vi "Main.vi"() -> ()   [LabVIEW 2021]
uses:
  Hamamatsu_class/SubRegion.ctl
  Application_class/Application.lvclass
  CetoniPump_class/CetoniPump.lvclass
  <vilib>/vision/Image Controls.llb/IMAQ Image.ctl
  Coriolis_Sim_class/Coriolis_Sim.lvclass
  C:/GIT/DensityGradientProject/CoriFlowBFS1Plus_class/CoriFlowBFS1Plus.lvclass
  CoriFlowBFS1Plus_class/CoriFlowBFS1Plus.lvclass
  Experiment_class/Experiment.lvclass
  <vilib>/Utility/error.llb/Error Cluster From Error Code.vi
  <vilib>/ErrorRing/Error Ring.xnode
  AD2_SDK_class/AD2_SDK.lvclass
  Hamamatsu_class/Hamamatsu.lvclass
panel:
  in  "Part of Experiment":bool
  in  "Numeric":dbl
  out "Configured Syringes":T1(array[cluster])
  in  "ABORT":bool
  out "Status":string="Cetoni Pump Initialized"
  out "Connected Pumps":T2(array[cluster])
  out "error out":errorcluster={"status"=TRUE, "code"=-2, "source"="labbCAN_Bus_API.lvlib:Error Converter (ErrCode or Status).vi<ERR>\nNo such entity\r\nThe given device config directory [C:\\Users\\Public\\Documents\\QmixElements\\Projects\\default_project\\Configurations] does not contain the required file device_properties.xml.\n\n\n<b>Complete call chain:</b>\r\n     labbCAN_Bus_API.lvlib:Error Converter (ErrCode or Status).vi\r\n     labbCAN_Bus_API.lvlib:LCB Open.vi\r\n     CetoniPump.lvclass:CetoniPump_Init.vi\r\n     Main.vi"}
  in  "Tab Control":T3(tab)=enum."LOG"
  in  "Connect TO Hardware":bool
  in  "Filter(0-1)Min-Max":dbl=0.5 min=0.0 max=1.0
  in  "Coriolis VISA resource name":refnum<visa-resource-name>="COM3"
  in  "Use Coriolis?":bool=TRUE
  in  "Cetoni Configuration Path":string="C:\\Users\\Public\\Documents\\QmixElements\\Projects\\default_project\\Configurations\\Gradient_generator_2"
  in  "Load and set latest":bool
  in  "Read Current Syringe \nConfiguration":bool
  in  "Read Continous":bool
  in  "Go to Level":bool
  in  "Go to Level":T4
  in  "index":i32
  in  "ReferenceMove":bool
  in  "ReadStatus":bool
  in  "ConfigureSyringe":bool
  in  "SyringeSettings":T5={"index"=0, "SyringeSettings"={"Maximum Piston Stroke (mm)"=100.0, "Inner Diameter (mm)"=12.0}}
  in  "Syringe (only for syringe helper)":T6(ring)=enum."BD 5ml"
  out "Syringe Helper":T7={"Maximum Piston Stroke (mm)"=48.147993421803335, "Inner Diameter (mm)"=12.06}
  in  "Stop ALL Pumps":bool
  in  "CetoniWaitData":T8
  in  "Cetoni Wait for Level":bool
  in  "Save Current Configuration":bool
  in  "Ramp IN flow":bool
  in  "Ramp In Settings":T9
  in  "Open Image Pairs Windows":bool
  in  "Open Live Window":bool
  in  "Center ROI":bool
  in  "Configure ROI":bool
  in  "ROI":T10={"Horizontal Offset"=0, "Vertical Offset"=0, "Horizontal Size"=2048, "Vertical Size"=2048} {"Vertical Size" min=4 max=2304 step=4; "Horizontal Size" min=4 max=2304 step=4; "Vertical Offset" min=0 max=0 step=4; "Horizontal Offset" min=0 max=0 step=4}
  in  "Go Live":bool
  in  "Set Exposure Time":bool
  in  "Read Redout Time":bool
  out "ReadoutTime":dbl
  in  "Exposure (ms)":dbl=5.0 step=1.0
  in  "Take HW Timed Image Pair":bool
  in  "Save HW Timed Image Pair":bool
  in  "Image Continously":bool
  in  "Configure Triggering":bool
  in  "Open DIO signal helper":bool
  in  "Triggering":T11={"Pulse Length(ms)"=10.0, "DIO0Offset(ms)"=0.0, "DIO1 Pulse time (ms)"=10.0, "DIO2 Pulse time (ms) 2"=100.0, "DIO3 Pulse time (ms) 3"=0.0, "EnableDIO3"=FALSE, "EnableDIO2"=TRUE, "EnableDIO1"=TRUE}
  out "Waveform Chart":T12(graph)
  in  "Read Continously?":bool
  in  "Read Coriolis":bool
  in  "Read Coriolis Buffer":bool
  out "Buffer":T13(array[cluster])
  out "Coriolis  Data":T14
  in  "Wait":bool
  in  "Wait":T15={"Wait Time"=0.0, "Reset"=FALSE, "Part of Experiment"=TRUE}
  in  "Read Trigges Values From HW Timed TAB":bool
  in  "Run Experiment":bool
  in  "Create Experiment":bool
  in  "Experiment Base path":path
  in  "Number of Images at each Level":u16
  in  "Levels (uL)":dbl[](array[numeric])
  in  "Triggering for experiment":T11
  in  "Ramp In (Experiment)":T9
  out "LOG":string
  in  "Exit":bool
  in  "Inject Error<Replace Me>":bool
  # "Not implemented"
  # "DIO0 Pulses at the same time as DIO1,2 and 3 +-offset"
  # "DIO0 Pulses at the same time as DIO1,2 \nand 3 +-offset"
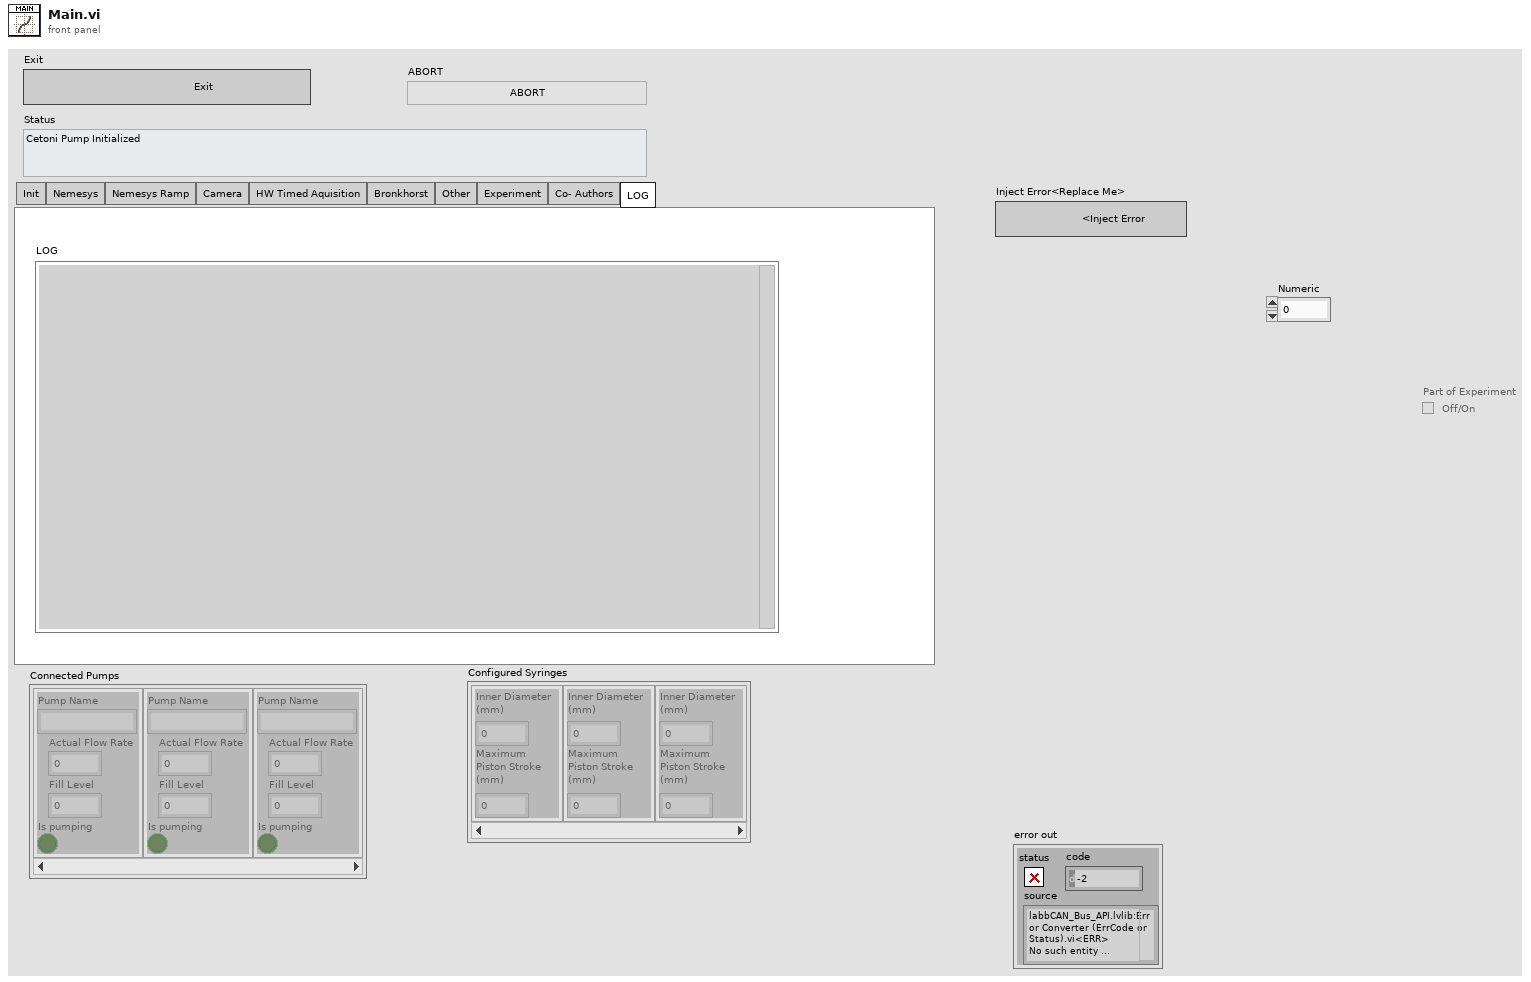
[diagram p1: front panel]
types:
  T1 = cluster{"Inner Diameter \n(mm)":dbl, "Maximum \nPiston Stroke \n(mm)":dbl}[]
  T2 = cluster{"Pump Name":string, "Actual Flow Rate":dbl, "Fill Level":dbl, "Is pumping":bool}[]
  T3 = enum32{"Init", "Nemesys", "Nemesys Ramp", "Camera", "HW Timed Aquisition", "Bronkhorst", "Other", "Experiment", "Co- Authors", "LOG"}
  T4 = cluster{"index":i32, "Flow (ul/min)":dbl, "Level(uL)":dbl}
  T5 = cluster{"index":i32, "SyringeSettings":cluster{"Maximum Piston Stroke (mm)":dbl, "Inner Diameter (mm)":dbl}}
  T6 = enum16{"BD 1ml", "BD 3ml", "BD 5ml", "BD 10ml", "BD 20ml", "BD 30ml", "BD 50ml", "HSW 1ml"}
  T7 = cluster{"Maximum Piston Stroke (mm)":dbl, "Inner Diameter (mm)":dbl}
  T8 = cluster{"Index":u8, "WaitCondition":enum16{"GE", "LE", "Stopped"}, "Value (uL)":dbl, "Experiment":bool}
  T9 = cluster{"Pump Controller":cluster{"Index of Pump Controller":u8, "Medium Start Before  Level (uL))":dbl, "Slow Start Before  Level (uL)":dbl, "Target Level (uL)":dbl}, "Pump Flows":cluster{"Index of Pump":u8, "Fast Flow":dbl, "Medium Flow":dbl, "Slow Flow":dbl}[]}
  T10 = typedef "Hamamatsu.lvclass/SubRegion.ctl" = cluster{"Horizontal Offset":i32, "Vertical Offset":i32, "Horizontal Size":i32, "Vertical Size":i32}
  T11 = cluster{"Pulse Length(ms)":dbl, "DIO0Offset(ms)":dbl, "DIO1 Pulse time (ms)":dbl, "DIO2 Pulse time (ms) 2":dbl, "DIO3 Pulse time (ms) 3":dbl, "EnableDIO3":bool, "EnableDIO2":bool, "EnableDIO1":bool}
  T12 = cluster{"Density_g_L":sgl, "FLow(ul/min)":sgl, "Temperature(C)":sgl}
  T13 = cluster{"Cluster":cluster{"Density_g_L":sgl, "FLow(ul/min)":sgl, "Temperature(C)":sgl}, "current time":timestamp}[]
  T14 = cluster{"Cluster":cluster{"Density_g_L":sgl, "FLow(ul/min)":sgl, "Temperature(C)":sgl}, "current time":timestamp}
  T15 = cluster{"Wait Time":dbl, "Reset":bool, "Part of Experiment":bool}
  T16 = enum8{"Enabled", "Disabled", "Disabled and Grayed Out"}
  T17 = cluster{"Index":u8, "WaitCondition":enum16{"GE", "LE", "Stopped"}, "Value":dbl, "Experiment":bool}
  T18 = cluster{"Pump Handle":i64, "Pump Name":string, "Maximum Volume":dbl, "Maximum Flow Rate":dbl, "Flow Rate":dbl, "Target Level":dbl}[]
  T19 = cluster{"Inner Diameter (mm)":dbl, "Maximum Piston Stroke (mm)":dbl}[]
  T20 = cluster{"Ramp In Settings":cluster{"Pump Controller":cluster{"Index of Pump Controller":u8, "Medium Start Before  Level (uL))":dbl, "Slow Start Before  Level (uL)":dbl, "Target Level (uL)":dbl}, "Pump Flows":cluster{"Index of Pump":u8, "Fast Flow":dbl, "Medium Flow":dbl, "Slow Flow":dbl}[]}, bool}
  T21 = cluster{"Fill Level":dbl, "Is pumping":bool, "Actual Flow Rate":dbl}
  T22 = typedef "IMAQ Image.ctl" = refnum<image>
  T23 = typedef "LVMinMaxIncTypeDef.ctl" = cluster{"Minimum":dbl, "Maximum":dbl, "Increment":dbl}
  T24 = cluster{"H Offset":cluster{"Value":i32, "Limits":T23}, "V Offset":cluster{"Value":i32, "Limits":T23}, "H Size":cluster{"Value":i32, "Limits":T23}, "V Size":cluster{"Value":i32, "Limits":T23}}
  T25 = typedef "Hamamatsu.lvclass/SubRegionLimits.ctl" = cluster{"H Offset":cluster{"Value":i32, "Limits":T23}, "V Offset":cluster{"Value":i32, "Limits":T23}, "H Size":cluster{"Value":i32, "Limits":T23}, "V Size":cluster{"Value":i32, "Limits":T23}}
  T26 = enum32{"Invalid", "Standard", "Closed", "Hidden", "Minimized", "Maximized"}
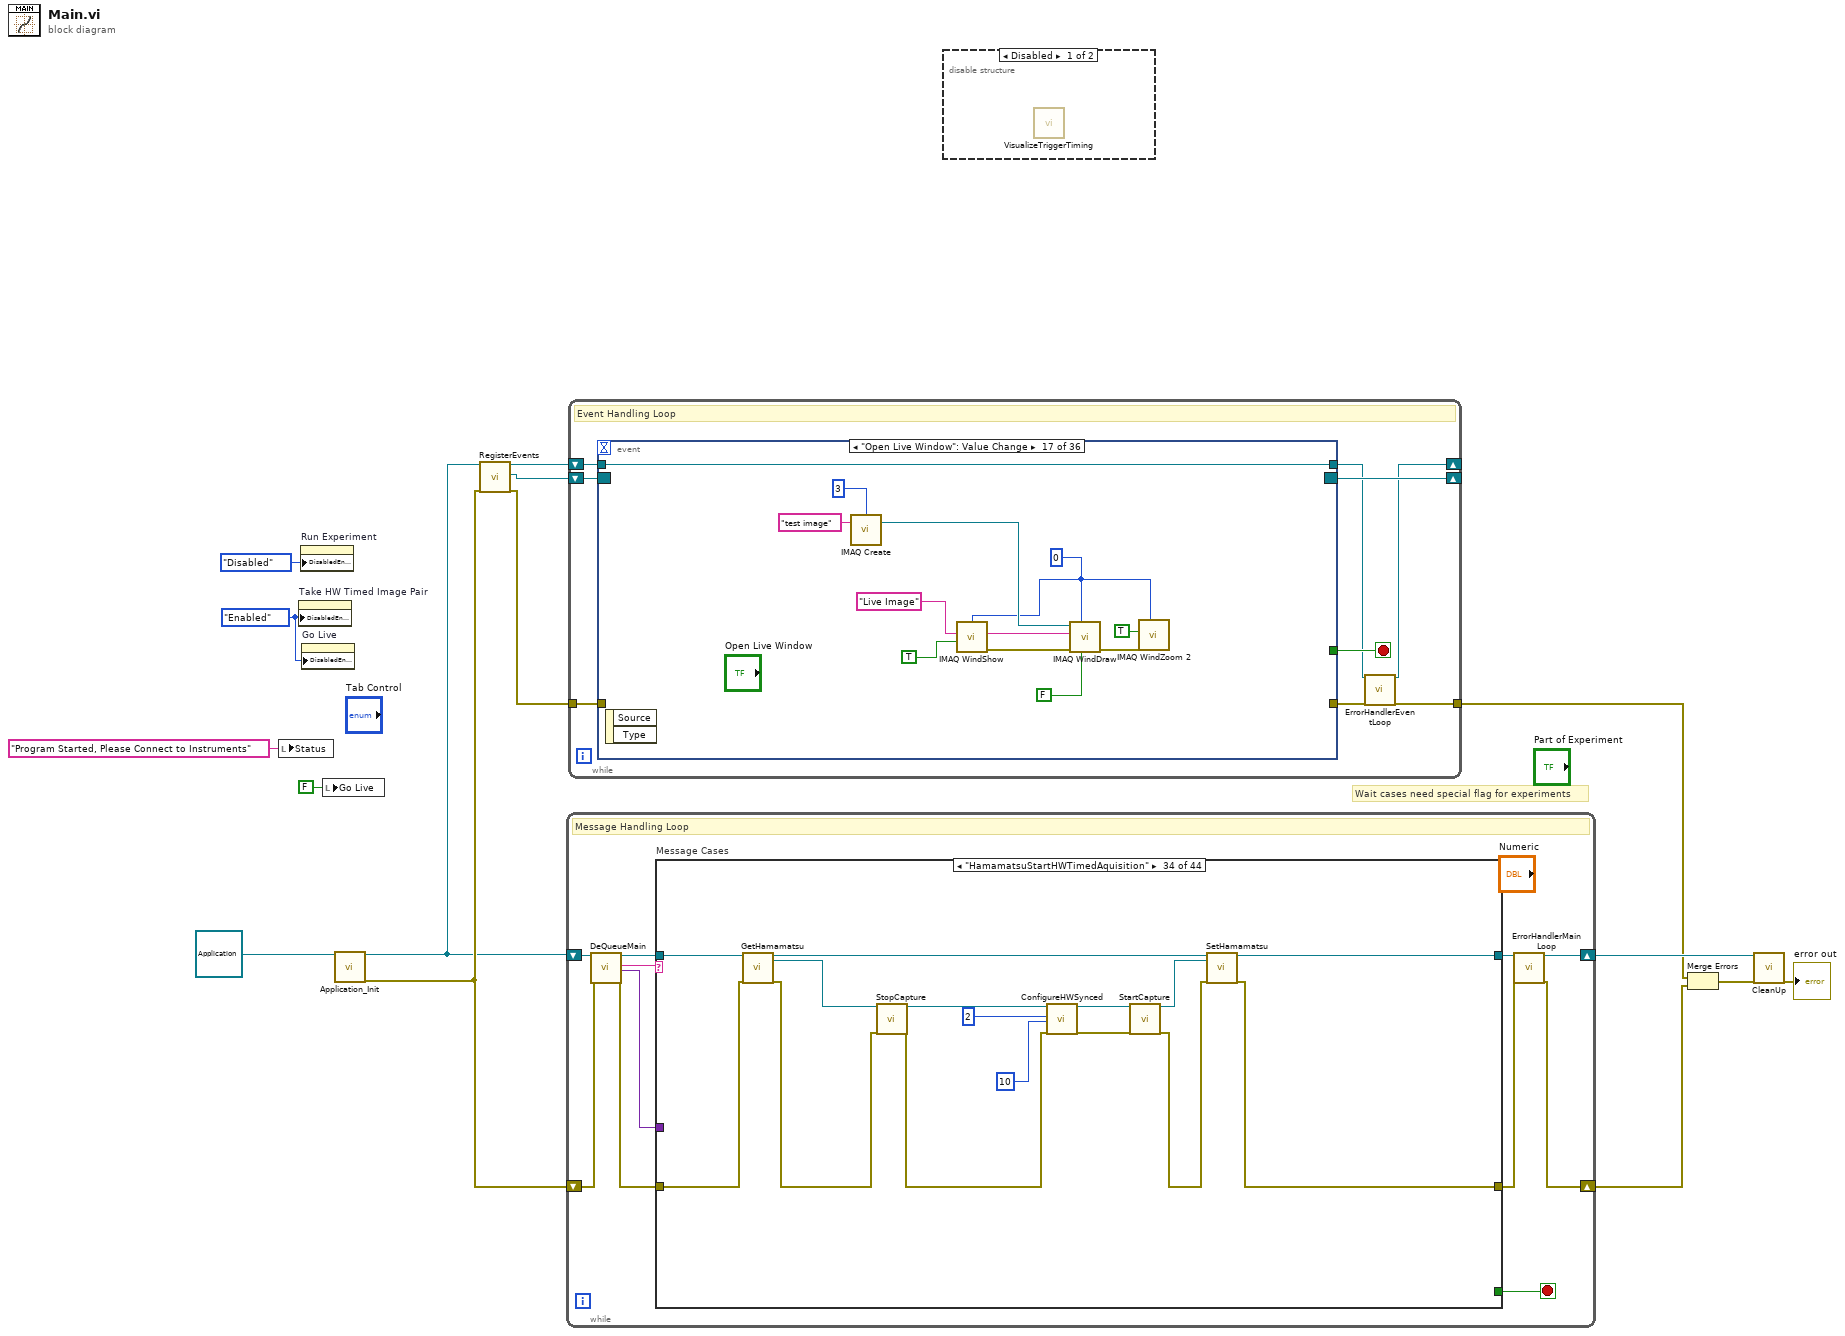
[diagram p0: block diagram]
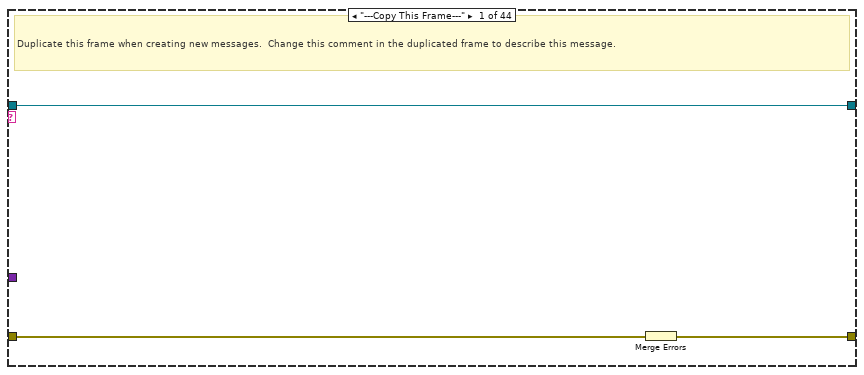
[diagram p3: hidden frame]
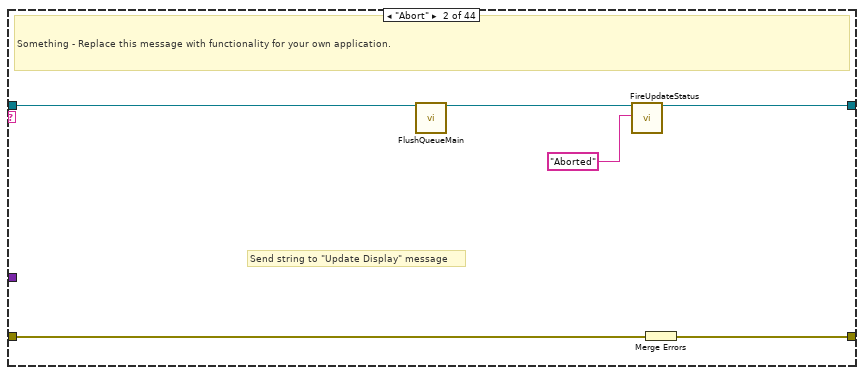
[diagram p4: hidden frame]
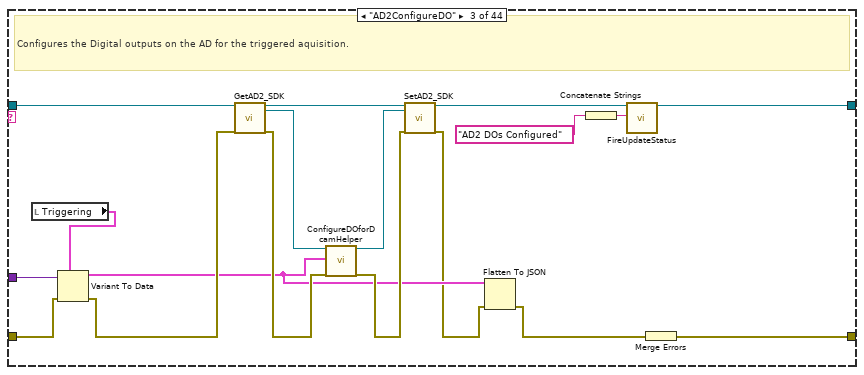
[diagram p5: hidden frame]
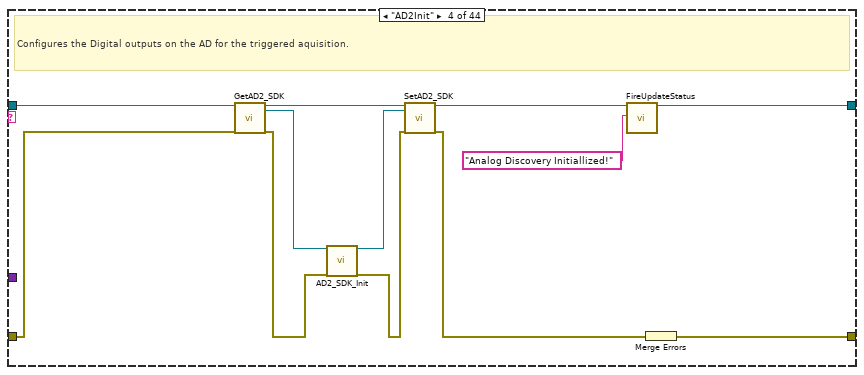
[diagram p6: hidden frame]
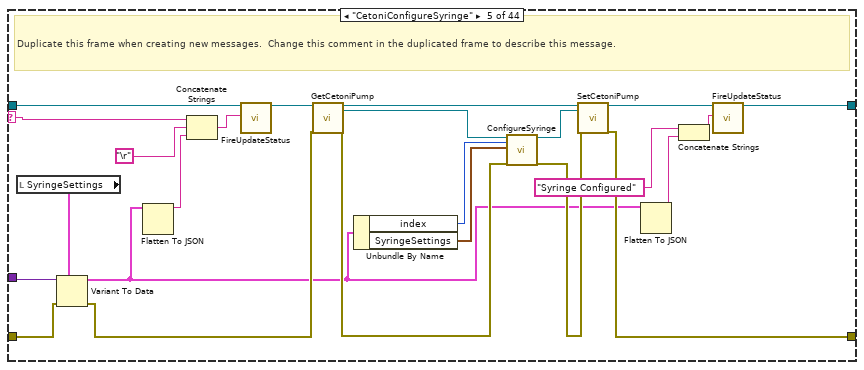
[diagram p7: hidden frame]
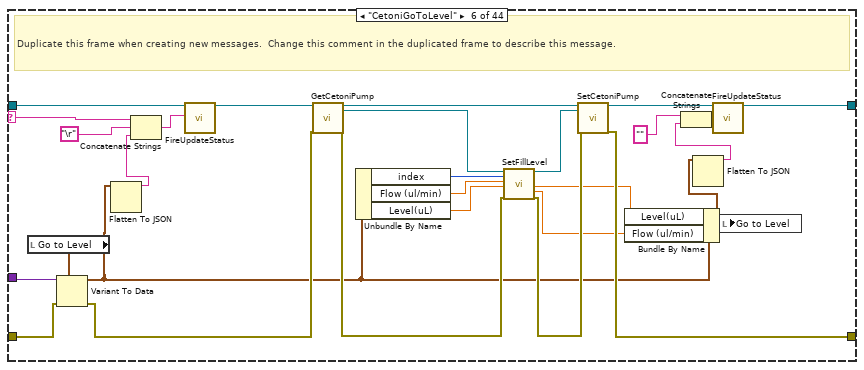
[diagram p8: hidden frame]
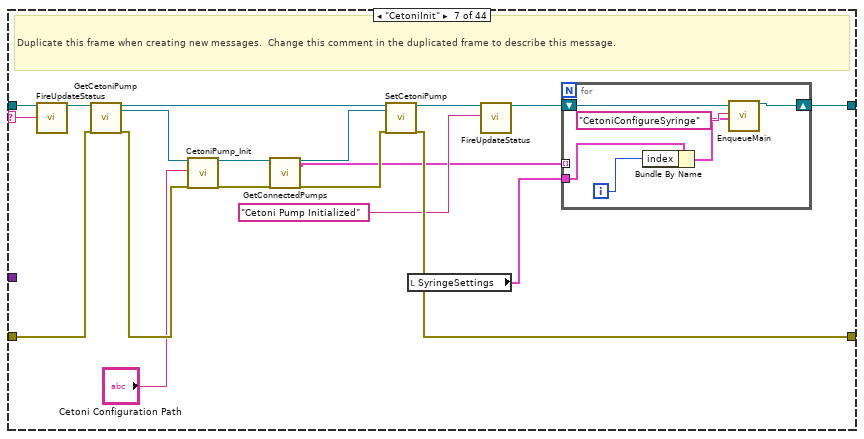
[diagram p9: hidden frame]
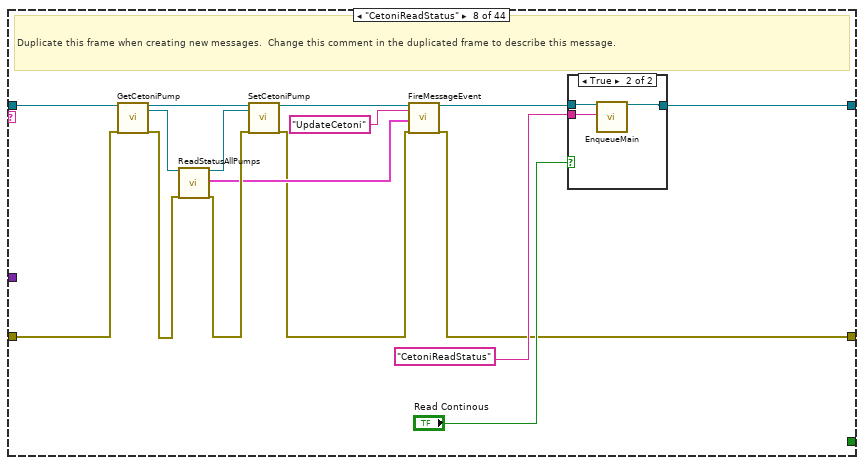
[diagram p10: hidden frame]
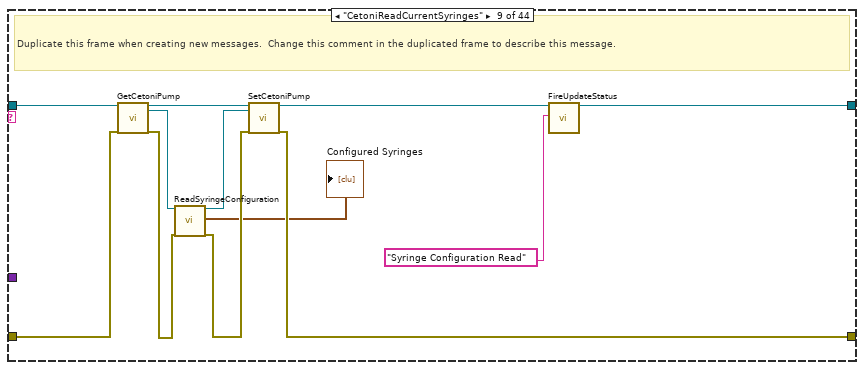
[diagram p12: hidden frame]
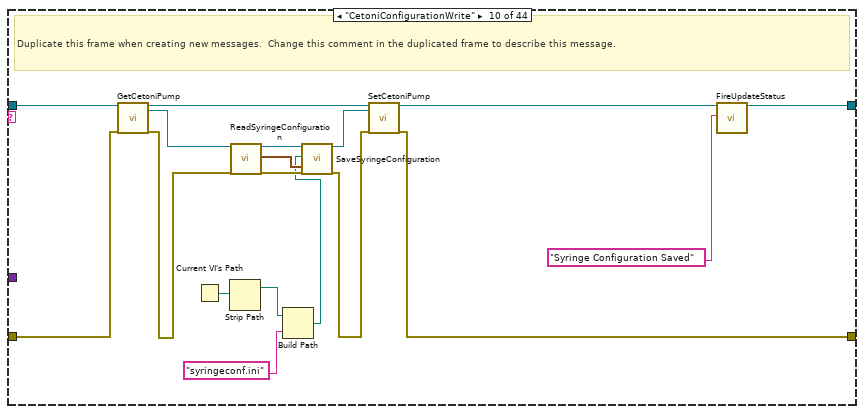
[diagram p13: hidden frame]
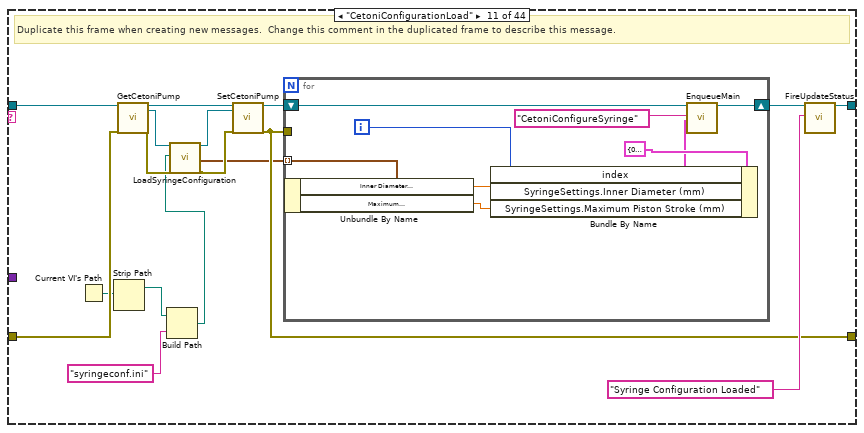
[diagram p14: hidden frame]
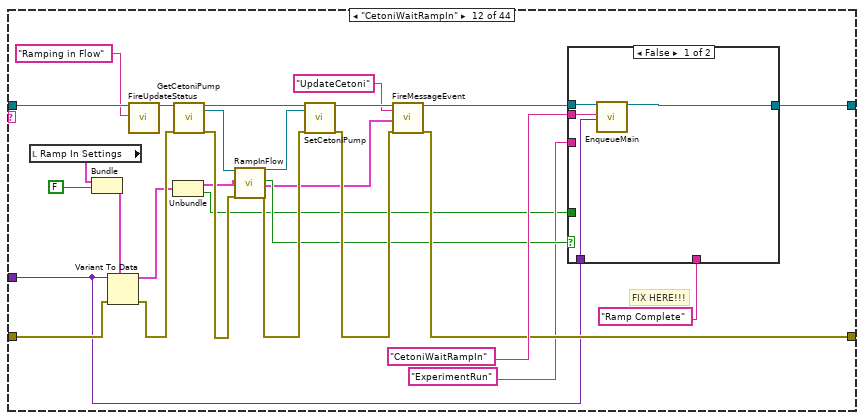
[diagram p15: hidden frame]
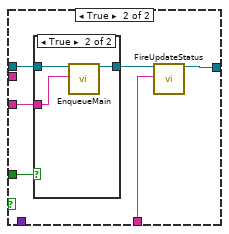
[diagram p16: hidden frame]
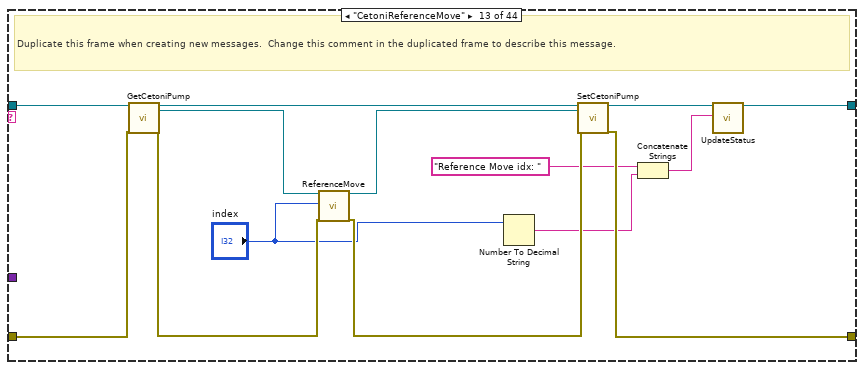
[diagram p18: hidden frame]
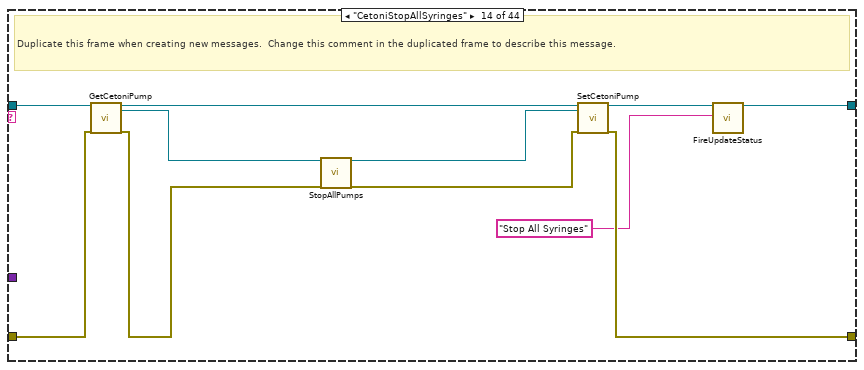
[diagram p19: hidden frame]
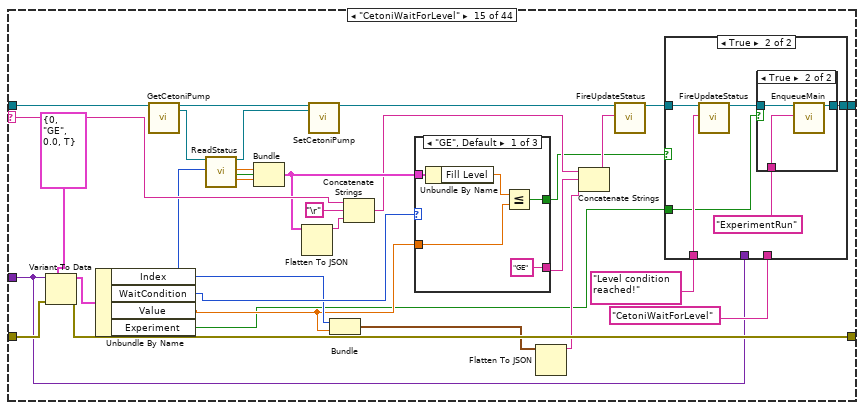
[diagram p20: hidden frame]
diagram:
  w3 = T16."Enabled" ("Disabled")
  # "Wait cases need special flag for experiments"
  n1 = local write "Status"("Program Started, Please Connect to Instruments" ("Status")) -> ()
  n2 = property on="Take HW Timed Image Pair" class="Bool"("DisabledEnum"=w3) -> ()  [unwired: 2 in, 2 out]
  n3 = property on="Run Experiment" class="Bool"("DisabledEnum"=T16."Disabled" ("Disabled")) -> ()  [unwired: 2 in, 2 out]
  n4 = property on="Go Live" class="Bool (strict)"("DisabledEnum"=w3) -> ()  [unwired: 2 in, 2 out]
  n5 = local write "Go Live"(FALSE ("Go Live")) -> ()
  n6 = call "Application_Init.vi"("object in"=refnum<class "Application.lvclass"> refnum ("Application")) -> ("object out"=w5:refnum<class "Application.lvclass">, "error out"=w11:errorcluster)  [unwired: 17 in]
  n7 = call-dynamic "RegisterEvents.vi"("object in"=w5, "error in (no error)"=w11) -> ("object out"=w13:refnum<class "Application.lvclass">, "Event Registration Refnum"=w14:refnum<event-registration>, "error out"=w12:errorcluster)  [unwired: 15 in]
  n8 = while {
    shift-right: [w19] -> w10
    shift-left: w5 -> [w25]
    shift-right: [w20] -> w9
    shift-left: w11 -> [w16]
    stop <- w26 stop-if-true
    # "Message Handling Loop"
    n9 = call-dynamic "DeQueueMain.vi"("object in"=w25, "error in (no error)"=w16) -> ("object out"=w24:refnum<class "Application.lvclass">, "Message"=w23:string, "Message Data"=w22:variant, "error out"=w17:errorcluster)  [unwired: 14 in]
    n10 = case "Message Cases" shown="\"HamamatsuStartHWTimedAquisition\"" w23 {
      selector: w23 -> [_ _ _ _ w73 w103 w127 _ _ _ _ _ _ _ w311 _ _ _ _ _ _ _ _ _ _ _ _ _ _ _ _ w637 _ _ _ _ _ _ _ _ _ _ _ w872]
      tunnel: w17 -> [w29 w34 w43 w60 w84 w105 w134 w156 w172 w190 w207 w229 w270 w283 w306 w350 w361 w381 w401 w408 w417 w430 w432 w439 w466 w491 w507 w548 w571 w584 w616 w653 w662 w676 w693 w704 w731 w760 w765 w776 w814 w831 w843 _]
      tunnel: [w28 w35 w53 w65 w88 w115 w129 w143 w170 w188 w194 w236 w272 w281 w307 w349 w367 w393 w407 w409 w423 w425 w433 w448 w459 w491 w508 w554 w575 w583 w608 w652 w661 w674 w686 w702 w734 w760 w770 w797 w812 w832 w843 w873] -> w21
      tunnel: [_ _ _ _ _ _ _ _ _ _ _ _ _ _ _ _ _ _ _ _ _ _ TRUE _ _ _ _ _ _ _ _ _ _ _ _ _ _ _ _ _ _ _ _ _] -> w26
      tunnel: w22 -> [_ _ w45 _ w86 w99 _ _ _ _ _ w228 _ _ w289 _ _ _ _ _ _ w429 _ _ w468 _ _ _ _ _ _ _ _ _ _ _ _ _ w768 _ _ _ w844 _]
      tunnel: w24 -> [w27 w33 w50 w62 w71 w116 w135 w157 w173 w191 w208 w245 w273 w284 w316 w346 w366 w392 w406 w411 w422 w424 w434 w447 w470 w492 w516 w553 w574 w587 w617 w638 w665 w680 w696 w705 w727 w755 w769 w784 w815 w830 w846 w871]
      tunnel: [w27 w31 w41 w55 w70 w94 w124 w154 w164 w187 w205 w243 w265 w276 w292 w347 w356 w389 w404 w412 w419 w424 w435 w446 w455 w493 w515 w535 w556 w577 w611 w654 w663 w675 w687 w703 w737 w756 w769 w802 w805 w830 w845 w871] -> w18
      frame "---Copy This Frame---" {
        # "Duplicate this frame when creating new messages.  Change this comment in the duplicated frame to describe this message."
        n11 = Merge Errors(w29) -> (w28:errorcluster)
      }
      frame "Abort" {
        # "Send string to \"Update Display\" message"
        # "Something - Replace this message with functionality for your own application."
        n12 = call-dynamic "FlushQueueMain.vi"("object in"=w33) -> ("object out"=w32:refnum<class "Application.lvclass">)  [unwired: 16 in, 2 out]
        n13 = call-dynamic "FireUpdateStatus.vi"("object in"=w32, "Status"="Aborted") -> ("object out"=w31:refnum<class "Application.lvclass">)  [unwired: 16 in, 1 out]
        n14 = Merge Errors(w34) -> (w35:errorcluster)
      }
      frame "AD2ConfigureDO" {
        # "Configures the Digital outputs on the AD for the triggered aquisition."
        n15 = local read "Triggering"() -> (w42:T11)
        n16 = Variant To Data(error in=w43, type=w42, Variant=w45) -> (data=w39:T11, error out=w44:errorcluster)
        n17 = call-dynamic "GetAD2_SDK.vi"("object in"=w50, "error in (no error)"=w44) -> ("object out"=w52:refnum<class "Application.lvclass">, "AD2_SDK"=w47:refnum<class "AD2_SDK.lvclass">, "error out"=w49:errorcluster)  [unwired: 15 in]
        n18 = call-dynamic "ConfigureDOforDcamHelper.vi"("object in"=w47, "Pulse Settings"=w39, "error in (no error)"=w49) -> ("object out"=w46:refnum<class "AD2_SDK.lvclass">, "error out"=w48:errorcluster)  [unwired: 15 in]
        n19 = call-dynamic "SetAD2_SDK.vi"("object in"=w52, "AD2_SDK"=w46, "error in (no error)"=w48) -> ("object out"=w51:refnum<class "Application.lvclass">, "error out"=w38:errorcluster)  [unwired: 15 in]
        n20 = Flatten To JSON(anything=w39, error in (no error)=w38) -> (11:w37:errorcluster)  [unwired: 1 in, 1 out]
        n21 = Concatenate Strings("AD2 DOs Configured" ("Status")) -> (w36:string)
        n22 = call-dynamic "FireUpdateStatus.vi"("object in"=w51, "Status"=w36) -> ("object out"=w41:refnum<class "Application.lvclass">)  [unwired: 16 in, 1 out]
        n23 = Merge Errors(w37) -> (w53:errorcluster)
      }
      frame "AD2Init" {
        # "Configures the Digital outputs on the AD for the triggered aquisition."
        n24 = call-dynamic "GetAD2_SDK.vi"("object in"=w62, "error in (no error)"=w60) -> ("object out"=w64:refnum<class "Application.lvclass">, "AD2_SDK"=w59:refnum<class "AD2_SDK.lvclass">, "error out"=w57:errorcluster)  [unwired: 15 in]
        n25 = call "AD2_SDK_Init.vi"("object in"=w59, "error in (no error)"=w57) -> ("object out"=w58:refnum<class "AD2_SDK.lvclass">, "error out"=w56:errorcluster)  [unwired: 16 in]
        n26 = call-dynamic "SetAD2_SDK.vi"("object in"=w64, "AD2_SDK"=w58, "error in (no error)"=w56) -> ("object out"=w63:refnum<class "Application.lvclass">, "error out"=w61:errorcluster)  [unwired: 15 in]
        n27 = call-dynamic "FireUpdateStatus.vi"("object in"=w63, "Status"="Analog Discovery Initiallized!") -> ("object out"=w55:refnum<class "Application.lvclass">)  [unwired: 16 in, 1 out]
        n28 = Merge Errors(w61) -> (w65:errorcluster)
      }
      frame "CetoniConfigureSyringe" {
        # "Duplicate this frame when creating new messages.  Change this comment in the duplicated frame to describe this message."
        n29 = local read "SyringeSettings"() -> (w79:T5)
        n30 = Variant To Data(error in=w84, type=w79, Variant=w86) -> (data=w67:T5, error out=w85:errorcluster)
        n31 = Flatten To JSON(anything=w67) -> (JSON string=w74:string)  [unwired: 2 in, 1 out]
        n32 = Concatenate Strings(w73, "\r", w74) -> (w75:string)
        n33 = call-dynamic "FireUpdateStatus.vi"("object in"=w71, "Status"=w75) -> ("object out"=w72:refnum<class "Application.lvclass">)  [unwired: 16 in, 1 out]
        n34 = call-dynamic "GetCetoniPump.vi"("object in"=w72, "error in (no error)"=w85) -> ("object out"=w89:refnum<class "Application.lvclass">, "CetoniPump"=w81:refnum<class "CetoniPump.lvclass">, "error out"=w83:errorcluster)  [unwired: 15 in]
        n35 = Unbundle By Name(w67) -> ("index"=w78:i32, "SyringeSettings"=w77:T7)
        n36 = call-dynamic "ConfigureSyringe.vi"("object in"=w81, "index"=w78, "SyringeSettings"=w77, "error in (no error)"=w83) -> ("object out"=w80:refnum<class "CetoniPump.lvclass">, "error out"=w82:errorcluster)  [unwired: 14 in]
        n37 = call-dynamic "SetCetoniPump.vi"("object in"=w89, "CetoniPump"=w80, "error in (no error)"=w82) -> ("object out"=w87:refnum<class "Application.lvclass">, "error out"=w88:errorcluster)  [unwired: 15 in]
        n38 = Flatten To JSON(anything=w67) -> (JSON string=w66:string)  [unwired: 2 in, 1 out]
        n39 = Concatenate Strings("Syringe Configured" ("Status"), w66) -> (w68:string)
        n40 = call-dynamic "FireUpdateStatus.vi"("object in"=w87, "Status"=w68) -> ("object out"=w70:refnum<class "Application.lvclass">)  [unwired: 16 in, 1 out]
      }
      frame "CetoniGoToLevel" {
        # "Duplicate this frame when creating new messages.  Change this comment in the duplicated frame to describe this message."
        n41 = local read "Go to Level"() -> (w104:T4)
        n42 = Variant To Data(error in=w105, type=w104, Variant=w99) -> (data=w97:T4, error out=w106:errorcluster)
        n43 = Flatten To JSON(anything=w97) -> (JSON string=w98:string)  [unwired: 2 in, 1 out]
        n44 = Concatenate Strings(w103, "\r", w98) -> (w100:string)
        n45 = call-dynamic "FireUpdateStatus.vi"("object in"=w116, "Status"=w100) -> ("object out"=w101:refnum<class "Application.lvclass">)  [unwired: 16 in, 1 out]
        n46 = call-dynamic "GetCetoniPump.vi"("object in"=w101, "error in (no error)"=w106) -> ("object out"=w117:refnum<class "Application.lvclass">, "CetoniPump"=w113:refnum<class "CetoniPump.lvclass">, "error out"=w111:errorcluster)  [unwired: 15 in]
        n47 = Unbundle By Name(w97) -> ("index"=w109:i32, "Flow (ul/min)"=w108:dbl, "Level(uL)"=w107:dbl)
        n48 = call-dynamic "SetFillLevel.vi"("object in"=w113, "index"=w109, "Flow"=w108, "Level(ml)"=w107, "error in (no error)"=w111) -> ("object out"=w112:refnum<class "CetoniPump.lvclass">, "Coerced Level"=w96:dbl, "Coerced Flow"=w95:dbl, "error out"=w110:errorcluster)  [unwired: 10 in, 1 out]
        n49 = call-dynamic "SetCetoniPump.vi"("object in"=w117, "CetoniPump"=w112, "error in (no error)"=w110) -> ("object out"=w114:refnum<class "Application.lvclass">, "error out"=w115:errorcluster)  [unwired: 15 in]
        n50 = Bundle By Name(cluster=w97, "Level(uL)"=w96, "Flow (ul/min)"=w95) -> (w91:T4)
        n51 = Flatten To JSON(anything=w91) -> (JSON string=w90:string)  [unwired: 2 in, 1 out]
        n52 = Concatenate Strings("" ("Status"), w90) -> (w92:string)
        n53 = call-dynamic "FireUpdateStatus.vi"("object in"=w114, "Status"=w92) -> ("object out"=w94:refnum<class "Application.lvclass">)  [unwired: 16 in, 1 out]
        n54 = local write "Go to Level"(w91) -> ()
      }
      frame "CetoniInit" {
        # "Duplicate this frame when creating new messages.  Change this comment in the duplicated frame to describe this message."
        n55 = call-dynamic "FireUpdateStatus.vi"("object in"=w135, "Status"=w127) -> ("object out"=w128:refnum<class "Application.lvclass">)  [unwired: 16 in, 1 out]
        n56 = call-dynamic "GetCetoniPump.vi"("object in"=w128, "error in (no error)"=w134) -> ("object out"=w136:refnum<class "Application.lvclass">, "CetoniPump"=w133:refnum<class "CetoniPump.lvclass">, "error out"=w132:errorcluster)  [unwired: 15 in]
        n57 = call "CetoniPump_Init.vi"("object in"=w133, "Device Configuration Path"="Cetoni Configuration Path", "error in (no error)"=w132) -> ("object out"=w123:refnum<class "CetoniPump.lvclass">, "error out"=w121:errorcluster)  [unwired: 15 in]
        n58 = call-dynamic "GetConnectedPumps.vi"("object in"=w123, "error in (no error)"=w121) -> ("object out"=w122:refnum<class "CetoniPump.lvclass">, "ConnectedPumps"=w119:T18, "error out"=w120:errorcluster)  [unwired: 15 in]
        n59 = call-dynamic "SetCetoniPump.vi"("object in"=w136, "CetoniPump"=w122, "error in (no error)"=w120) -> ("object out"=w130:refnum<class "Application.lvclass">, "error out"=w129:errorcluster)  [unwired: 15 in]
        n60 = local read "SyringeSettings"() -> (w118:T5)
        n61 = call-dynamic "FireUpdateStatus.vi"("object in"=w130, "Status"="Cetoni Pump Initialized") -> ("object out"=w126:refnum<class "Application.lvclass">)  [unwired: 16 in, 1 out]
        n62 = for {
          shift-right: [w141] -> w124
          shift-left: w126 -> [w142]
          tunnel: w119 -> [_] mode=indexing
          tunnel: w118 -> [w139]
          i -> [w138]
          n63 = Bundle By Name(cluster=w139, "index"=w138) -> (w137:T5)
          n64 = call-dynamic "EnqueueMain.vi"("object in"=w142, "Message"="CetoniConfigureSyringe", "Message Data"=w137) -> ("object out"=w141:refnum<class "Application.lvclass">)  [unwired: 15 in, 1 out]
        }
      }
      frame "CetoniReadStatus" {
        # "Duplicate this frame when creating new messages.  Change this comment in the duplicated frame to describe this message."
        n65 = call-dynamic "GetCetoniPump.vi"("object in"=w157, "error in (no error)"=w156) -> ("object out"=w158:refnum<class "Application.lvclass">, "CetoniPump"=w151:refnum<class "CetoniPump.lvclass">, "error out"=w150:errorcluster)  [unwired: 15 in]
        n66 = call-dynamic "ReadStatusAllPumps.vi"("object in"=w151, "error in (no error)"=w150) -> ("object out"=w148:refnum<class "CetoniPump.lvclass">, "Array"=w145:T2, "error out"=w149:errorcluster)  [unwired: 15 in]
        n67 = call-dynamic "SetCetoniPump.vi"("object in"=w158, "CetoniPump"=w148, "error in (no error)"=w149) -> ("object out"=w155:refnum<class "Application.lvclass">, "error out"=w144:errorcluster)  [unwired: 15 in]
        n68 = call-dynamic "FireMessageEvent.vi"("object in"=w155, "Message"="UpdateCetoni", "Message Data"=w145, "error in (no error)"=w144) -> ("object out"=w147:refnum<class "Application.lvclass">, "error out"=w143:errorcluster)  [unwired: 14 in]
        n69 = case shown="True" "Read Continous" {
          tunnel: w147 -> [w159 w162]
          tunnel: [w159 w161] -> w154
          tunnel: "CetoniReadStatus" ("Message") -> [_ w160]
          frame False {
          }
          frame True {
            n70 = call-dynamic "EnqueueMain.vi"("object in"=w162, "Message"=w160) -> ("object out"=w161:refnum<class "Application.lvclass">)  [unwired: 16 in, 1 out]
          }
        }
      }
      frame "CetoniReadCurrentSyringes" {
        # "Duplicate this frame when creating new messages.  Change this comment in the duplicated frame to describe this message."
        n71 = call-dynamic "GetCetoniPump.vi"("object in"=w173, "error in (no error)"=w172) -> ("object out"=w174:refnum<class "Application.lvclass">, "CetoniPump"=w169:refnum<class "CetoniPump.lvclass">, "error out"=w167:errorcluster)  [unwired: 15 in]
        n72 = call-dynamic "ReadSyringeConfiguration.vi"("object in"=w169, "error in (no error)"=w167) -> ("object out"=w168:refnum<class "CetoniPump.lvclass">, "COnfigured Syringes"=→"Configured Syringes":T19, "error out"=w166:errorcluster)  [unwired: 15 in]
        n73 = call-dynamic "SetCetoniPump.vi"("object in"=w174, "CetoniPump"=w168, "error in (no error)"=w166) -> ("object out"=w171:refnum<class "Application.lvclass">, "error out"=w170:errorcluster)  [unwired: 15 in]
        n74 = call-dynamic "FireUpdateStatus.vi"("object in"=w171, "Status"="Syringe Configuration Read") -> ("object out"=w164:refnum<class "Application.lvclass">)  [unwired: 16 in, 1 out]
      }
      frame "CetoniConfigurationWrite" {
        # "Duplicate this frame when creating new messages.  Change this comment in the duplicated frame to describe this message."
        n75 = call-dynamic "GetCetoniPump.vi"("object in"=w191, "error in (no error)"=w190) -> ("object out"=w192:refnum<class "Application.lvclass">, "CetoniPump"=w183:refnum<class "CetoniPump.lvclass">, "error out"=w179:errorcluster)  [unwired: 15 in]
        n76 = Current VI's Path() -> (path=w178:path)
        n77 = Strip Path(path=w178) -> (stripped path=w177:path)  [unwired: 1 out]
        n78 = call-dynamic "ReadSyringeConfiguration.vi"("object in"=w183, "error in (no error)"=w179) -> ("object out"=w182:refnum<class "CetoniPump.lvclass">, "COnfigured Syringes"=w181:T19, "error out"=w180:errorcluster)  [unwired: 15 in]
        n79 = Build Path(base path=w177, name or relative path="syringeconf.ini" ("Status")) -> (appended path=w175:path)
        n80 = call-dynamic "SaveSyringeConfiguration.vi"("object in"=w182, "configuration file in"=w175, "Write"=w181, "error in (no error)"=w180) -> ("object out"=w184:refnum<class "CetoniPump.lvclass">, "error out"=w185:errorcluster)  [unwired: 14 in]
        n81 = call-dynamic "SetCetoniPump.vi"("object in"=w192, "CetoniPump"=w184, "error in (no error)"=w185) -> ("object out"=w189:refnum<class "Application.lvclass">, "error out"=w188:errorcluster)  [unwired: 15 in]
        n82 = call-dynamic "FireUpdateStatus.vi"("object in"=w189, "Status"="Syringe Configuration Saved") -> ("object out"=w187:refnum<class "Application.lvclass">)  [unwired: 16 in, 1 out]
      }
      frame "CetoniConfigurationLoad" {
        # "Duplicate this frame when creating new messages.  Change this comment in the duplicated frame to describe this message."
        n83 = Current VI's Path() -> (path=w203:path)
        n84 = Strip Path(path=w203) -> (stripped path=w202:path)  [unwired: 1 out]
        n85 = call-dynamic "GetCetoniPump.vi"("object in"=w208, "error in (no error)"=w207) -> ("object out"=w209:refnum<class "Application.lvclass">, "CetoniPump"=w200:refnum<class "CetoniPump.lvclass">, "error out"=w199:errorcluster)  [unwired: 15 in]
        n86 = Build Path(base path=w202, name or relative path="syringeconf.ini" ("Status")) -> (appended path=w198:path)
        n87 = call-dynamic "LoadSyringeConfiguration.vi"("object in"=w200, "configuration file path"=w198, "error in (no error)"=w199) -> ("object out"=w197:refnum<class "CetoniPump.lvclass">, "Read 2"=w193:T1, "error out"=w196:errorcluster)  [unwired: 13 in, 1 out]
        n88 = call-dynamic "SetCetoniPump.vi"("object in"=w209, "CetoniPump"=w197, "error in (no error)"=w196) -> ("object out"=w206:refnum<class "Application.lvclass">, "error out"=w194:errorcluster)  [unwired: 15 in]
        n89 = for {
          shift-right: [w216] -> w195
          shift-left: w206 -> [w218]
          tunnel: w194 -> [_]
          tunnel: w193 -> [w212] mode=indexing
          i -> [w215]
          n90 = Unbundle By Name(w212) -> ("Inner Diameter \n(mm)"=w211:dbl, "Maximum \nPiston Stroke \n(mm)"=w210:dbl)
          n91 = Bundle By Name(cluster=T5 {"index"=0, "SyringeSettings"={"Maximum Piston Stroke (mm)"=100.0, "Inner Diameter (mm)"=12.0}} ("SyringeSettings 2"), "index"=w215, "SyringeSettings.Inner Diameter (mm)"=w211, "SyringeSettings.Maximum Piston Stroke (mm)"=w210) -> (w214:T5)
          n92 = call-dynamic "EnqueueMain.vi"("object in"=w218, "Message"="CetoniConfigureSyringe", "Message Data"=w214) -> ("object out"=w216:refnum<class "Application.lvclass">)  [unwired: 15 in, 1 out]
        }
        n93 = call-dynamic "FireUpdateStatus.vi"("object in"=w195, "Status"="Syringe Configuration Loaded") -> ("object out"=w205:refnum<class "Application.lvclass">)  [unwired: 16 in, 1 out]
      }
      frame "CetoniWaitRampIn" {
        # "FIX HERE!!!"
        n94 = local read "Ramp In Settings"() -> (w224:T9)
        n95 = Bundle("Ramp In Settings"=w224, FALSE) -> (w223:T20)  [unwired: 1 in]
        n96 = Variant To Data(error in=w229, type=w223, Variant=w228) -> (data=w220:T20, error out=w225:errorcluster)
        n97 = call-dynamic "FireUpdateStatus.vi"("object in"=w245, "Status"="Ramping in Flow" ("Message")) -> ("object out"=w235:refnum<class "Application.lvclass">)  [unwired: 16 in, 1 out]
        n98 = Unbundle(w220) -> ("Ramp In Settings"=w221:T9, w219:bool)
        n99 = call-dynamic "GetCetoniPump.vi"("object in"=w235, "error in (no error)"=w225) -> ("object out"=w246:refnum<class "Application.lvclass">, "CetoniPump"=w241:refnum<class "CetoniPump.lvclass">, "error out"=w240:errorcluster)  [unwired: 15 in]
        n100 = call-dynamic "RampInFlow.vi"("object in"=w241, "Ramp In Settings"=w221, "error in (no error)"=w240) -> ("object out"=w233:refnum<class "CetoniPump.lvclass">, "Target Level Reached"=w231:bool, "Pump Status out"=w227:T2, "error out"=w232:errorcluster)  [unwired: 13 in]
        n101 = call-dynamic "SetCetoniPump.vi"("object in"=w246, "CetoniPump"=w233, "error in (no error)"=w232) -> ("object out"=w244:refnum<class "Application.lvclass">, "error out"=w237:errorcluster)  [unwired: 15 in]
        n102 = call-dynamic "FireMessageEvent.vi"("object in"=w244, "Message"="UpdateCetoni", "Message Data"=w227, "error in (no error)"=w237) -> ("object out"=w239:refnum<class "Application.lvclass">, "error out"=w236:errorcluster)  [unwired: 14 in]
        n103 = case shown="False" w231 {
          tunnel: w239 -> [w250 w255]
          tunnel: [w249 w256] -> w243
          tunnel: "CetoniWaitRampIn" ("Message") -> [w248 _]
          tunnel: "Ramp Complete" ("Status") -> [_ w254]
          tunnel: w228 -> [w247 _]
          tunnel: "ExperimentRun" ("Message") -> [_ w252]
          tunnel: w219 -> [_ w251]
          frame False {
            n104 = call-dynamic "EnqueueMain.vi"("object in"=w250, "Message"=w248, "Message Data"=w247) -> ("object out"=w249:refnum<class "Application.lvclass">)  [unwired: 15 in, 1 out]
          }
          frame True {
            n105 = case shown="True" w251 {
              tunnel: w255 -> [w257 w260]
              tunnel: [w257 w259] -> w253
              tunnel: w252 -> [_ w258]
              frame False {
              }
              frame True {
                n106 = call-dynamic "EnqueueMain.vi"("object in"=w260, "Message"=w258) -> ("object out"=w259:refnum<class "Application.lvclass">)  [unwired: 16 in, 1 out]
              }
            }
            n107 = call-dynamic "FireUpdateStatus.vi"("object in"=w253, "Status"=w254) -> ("object out"=w256:refnum<class "Application.lvclass">)  [unwired: 16 in, 1 out]
          }
        }
      }
      frame "CetoniReferenceMove" {
        # "Duplicate this frame when creating new messages.  Change this comment in the duplicated frame to describe this message."
        n108 = call-dynamic "GetCetoniPump.vi"("object in"=w273, "error in (no error)"=w270) -> ("object out"=w274:refnum<class "Application.lvclass">, "CetoniPump"=w269:refnum<class "CetoniPump.lvclass">, "error out"=w267:errorcluster)  [unwired: 15 in]
        n109 = call-dynamic "ReferenceMove.vi"("object in"=w269, "index"="index", "error in (no error)"=w267) -> ("object out"=w268:refnum<class "CetoniPump.lvclass">, "error out"=w266:errorcluster)  [unwired: 15 in]
        n110 = Number To Decimal String(number="index") -> (decimal integer string=w261:string)  [unwired: 1 in]
        n111 = call-dynamic "SetCetoniPump.vi"("object in"=w274, "CetoniPump"=w268, "error in (no error)"=w266) -> ("object out"=w271:refnum<class "Application.lvclass">, "error out"=w272:errorcluster)  [unwired: 15 in]
        n112 = Concatenate Strings("Reference Move idx: " ("Status"), w261) -> (w263:string)
        n113 = call-dynamic "UpdateStatus.vi"("object in"=w271, "Status"=w263) -> ("object out"=w265:refnum<class "Application.lvclass">)  [unwired: 16 in, 1 out]
      }
      frame "CetoniStopAllSyringes" {
        # "Duplicate this frame when creating new messages.  Change this comment in the duplicated frame to describe this message."
        n114 = call-dynamic "GetCetoniPump.vi"("object in"=w284, "error in (no error)"=w283) -> ("object out"=w285:refnum<class "Application.lvclass">, "CetoniPump"=w278:refnum<class "CetoniPump.lvclass">, "error out"=w280:errorcluster)  [unwired: 15 in]
        n115 = call-dynamic "StopAllPumps.vi"("object in"=w278, "error in (no error)"=w280) -> ("object out"=w277:refnum<class "CetoniPump.lvclass">, "error out"=w279:errorcluster)  [unwired: 16 in]
        n116 = call-dynamic "SetCetoniPump.vi"("object in"=w285, "CetoniPump"=w277, "error in (no error)"=w279) -> ("object out"=w282:refnum<class "Application.lvclass">, "error out"=w281:errorcluster)  [unwired: 15 in]
        n117 = call-dynamic "FireUpdateStatus.vi"("object in"=w282, "Status"="Stop All Syringes") -> ("object out"=w276:refnum<class "Application.lvclass">)  [unwired: 16 in, 1 out]
      }
      frame "CetoniWaitForLevel" {
        n118 = Variant To Data(error in=w306, type=T17 {"Index"=0, "WaitCondition"=enum."GE", "Value"=0.0, "Experiment"=TRUE} ("CetoniWaitData"), Variant=w289) -> (data=w305:T17, error out=w307:errorcluster)
        n119 = Unbundle By Name(w305) -> ("Index"=w296:u8, "WaitCondition"=w304:enum16{"GE", "LE", "Stopped"}, "Value"=w295:dbl, "Experiment"=w286:bool)
        n120 = call-dynamic "GetCetoniPump.vi"("object in"=w316) -> ("object out"=w315:refnum<class "Application.lvclass">, "CetoniPump"=w314:refnum<class "CetoniPump.lvclass">)  [unwired: 16 in, 1 out]
        n121 = call-dynamic "ReadStatus.vi"("object in"=w314, "index"=w296) -> ("object out"=w313:refnum<class "CetoniPump.lvclass">, "Fill Level"=w310:dbl, "Is pumping"=w309:bool, "Actual Flow Rate"=w308:dbl)  [unwired: 13 in, 1 out]
        n122 = Bundle("Fill Level"=w310, "Is pumping"=w309, "Actual Flow Rate"=w308) -> (w303:T21)  [unwired: 1 in]
        n123 = Flatten To JSON(anything=w303) -> (JSON string=w300:string)  [unwired: 2 in, 1 out]
        n124 = call-dynamic "SetCetoniPump.vi"("object in"=w315, "CetoniPump"=w313) -> ("object out"=w302:refnum<class "Application.lvclass">)  [unwired: 16 in, 1 out]
        n125 = Bundle("Index"=w296, "Value"=w295) -> (w294:cluster{"Index":u8, "Value":dbl})  [unwired: 1 in]
        n126 = Concatenate Strings(w311, "\r", w300) -> (w299:string)
        n127 = case shown="\"GE\", Default" w304 {
          tunnel: w303 -> [w334 w340 w344]
          tunnel: w295 -> [w333 w338 _]
          tunnel: [w332 w337 w342] -> w291
          tunnel: ["GE" "LE" "Stopped"] -> w298
          frame "GE", Default {
            n128 = Unbundle By Name(w334) -> ("Fill Level"=w335:dbl)
            n129 = Less Or Equal?(x=w335, y=w333) -> (x <= y?=w332:bool)
          }
          frame "LE" {
            n130 = Unbundle By Name(w340) -> ("Fill Level"=w339:dbl)
            n131 = Less Or Equal?(x=w339, y=w338) -> (x <= y?=w337:bool)
          }
          frame "Stopped" {
            n132 = Unbundle By Name(w344) -> ("Is pumping"=w343:bool)
            n133 = Not(x=w343) -> (.not. x?=w342:bool)
          }
        }
        n134 = Flatten To JSON(anything=w294) -> (JSON string=w297:string)  [unwired: 2 in, 1 out]
        n135 = Concatenate Strings(w299, w298, w297) -> (w293:string)
        n136 = call-dynamic "FireUpdateStatus.vi"("object in"=w302, "Status"=w293) -> ("object out"=w301:refnum<class "Application.lvclass">)  [unwired: 16 in, 1 out]
        n137 = case shown="True" w291 {
          tunnel: w301 -> [w320 w325]
          tunnel: [w319 w323] -> w292
          tunnel: "CetoniWaitForLevel" ("Message") -> [w318 _]
          tunnel: w289 -> [w317 _]
          tunnel: "Level condition reached!" ("Status") -> [_ w324]
          tunnel: w286 -> [_ w322]
          frame False {
            n138 = call-dynamic "EnqueueMain.vi"("object in"=w320, "Message"=w318, "Message Data"=w317) -> ("object out"=w319:refnum<class "Application.lvclass">)  [unwired: 15 in, 1 out]
          }
          frame True {
            n139 = call-dynamic "FireUpdateStatus.vi"("object in"=w325, "Status"=w324) -> ("object out"=w326:refnum<class "Application.lvclass">)  [unwired: 16 in, 1 out]
            n140 = case shown="True" w322 {
              tunnel: w326 -> [w327 w330]
              tunnel: [w327 w329] -> w323
              tunnel: "ExperimentRun" ("Message") -> [_ w328]
              frame False {
              }
              frame True {
                n141 = call-dynamic "EnqueueMain.vi"("object in"=w330, "Message"=w328) -> ("object out"=w329:refnum<class "Application.lvclass">)  [unwired: 16 in, 1 out]
              }
            }
          }
        }
      }
      frame "Confirm Quit" {
        # "#CodeNeeded - If you want to provide an \"Are you sure\" dialog (or some other notification) before the application exits, place that code here. This message is typically sent from a Panel Close? event."
        # "Confirm Quit - Message that can confirm whether or not the user wants to exit the application."
        n142 = call-dynamic "EnqueueMain.vi"("object in"=w346, "Message"="Exit", "error in (no error)"=w350, "Priority Message? (F)"=TRUE) -> ("object out"=w347:refnum<class "Application.lvclass">, "error out"=w349:errorcluster)  [unwired: 14 in]
      }
      frame "CoriolisInit" {
        n143 = call-dynamic "GetCoriFlowBFS1Plus.vi"("object in"=w366) -> ("object out"=w365:refnum<class "Application.lvclass">, "CoriFlowBFS1Plus"=w363:refnum<class "CoriFlowBFS1Plus.lvclass">)  [unwired: 16 in, 1 out]
        n144 = case shown="True" "Use Coriolis?" {
          tunnel: [w371 w378] -> w352
          tunnel: w363 -> [_ _]
          tunnel: w361 -> [w369 w377]
          tunnel: [w368 w376] -> w354
          tunnel: "Coriolis VISA resource name" -> [_ w374]
          tunnel: "Filter(0-1)Min-Max" -> [_ w373]
          frame False {
            n145 = call "Coriolis_Sim_Init.vi"("object in"=refnum<class "Coriolis_Sim.lvclass"> refnum ("Coriolis_Sim"), "error in (no error)"=w369) -> ("object out"=w371:refnum<class "Coriolis_Sim.lvclass">, "error out"=w368:errorcluster)  [unwired: 16 in]
          }
          frame True {
            n146 = call "CoriFlowBFS1Plus_Init.vi"("object in"=refnum<class "CoriFlowBFS1Plus.lvclass"> refnum ("CoriFlowBFS1Plus"), "VISA resource name"=w374, "Filter(0-1)Min-Max"=w373, "SW Buffer Size"=1000, "error in (no error)"=w377) -> ("object out"=w378:refnum<class "CoriFlowBFS1Plus.lvclass">, "error out"=w376:errorcluster)  [unwired: 13 in]
          }
        }
        n147 = call-dynamic "SendZero.vi"("object in"=w352, "error in (no error)"=w354) -> ("object out"=w351:refnum<class "CoriFlowBFS1Plus.lvclass">, "error out"=w353:errorcluster)  [unwired: 16 in]
        n148 = call-dynamic "FireUpdateStatus.vi"("object in"=w365, "Status"="Zeroing Coriolis") -> ("object out"=w358:refnum<class "Application.lvclass">)  [unwired: 16 in, 1 out]
        n149 = call-dynamic "SetCoriFlowBFS1Plus.vi"("object in"=w358, "CoriFlowBFS1Plus"=w351) -> ("object out"=w364:refnum<class "Application.lvclass">)  [unwired: 16 in, 1 out]
        n150 = call-dynamic "FireUpdateStatus.vi"("object in"=w364, "Status"="Coriolis Initialized!") -> ("object out"=w356:refnum<class "Application.lvclass">)  [unwired: 16 in, 1 out]
        n151 = Merge Errors(w353) -> (w367:errorcluster)
      }
      frame "CoriolisMeasure" {
        # "Duplicate this frame when creating new messages.  Change this comment in the duplicated frame to describe this message."
        n152 = call-dynamic "GetCoriFlowBFS1Plus.vi"("object in"=w392) -> ("object out"=w391:refnum<class "Application.lvclass">, "CoriFlowBFS1Plus"=w383:refnum<class "CoriFlowBFS1Plus.lvclass">)  [unwired: 16 in, 1 out]
        n153 = call-dynamic "ReadLatest.vi"("object in"=w383, "error in (no error)"=w381) -> ("object out"=w382:refnum<class "CoriFlowBFS1Plus.lvclass">, "Latest Data"=w379:T14, "error out"=w380:errorcluster)  [unwired: 15 in]
        n154 = call-dynamic "SetCoriFlowBFS1Plus.vi"("object in"=w391, "CoriFlowBFS1Plus"=w382) -> ("object out"=w390:refnum<class "Application.lvclass">)  [unwired: 16 in, 1 out]
        n155 = call-dynamic "FireMessageEvent.vi"("object in"=w390, "Message"="UpdateCoriolis", "Message Data"=w379, "error in (no error)"=w380) -> ("object out"=w386:refnum<class "Application.lvclass">, "error out"=w384:errorcluster)  [unwired: 14 in]
        n156 = Merge Errors(w384) -> (w393:errorcluster)
        n157 = case shown="True" "Read Continously?" {
          tunnel: w386 -> [w394 w398]
          tunnel: [w394 w397] -> w389
          tunnel: "CoriolisMeasure" ("Message") -> [_ w396]
          frame False {
          }
          frame True {
            n158 = call-dynamic "EnqueueMain.vi"("object in"=w398, "Message"=w396, "Priority Message? (F)"=FALSE) -> ("object out"=w397:refnum<class "Application.lvclass">)  [unwired: 15 in, 1 out]
          }
        }
      }
      frame "CoriolisReadBuffer" {
        # "Duplicate this frame when creating new messages.  Change this comment in the duplicated frame to describe this message."
        n159 = call-dynamic "GetCoriFlowBFS1Plus.vi"("object in"=w406) -> ("object out"=w405:refnum<class "Application.lvclass">, "CoriFlowBFS1Plus"=w403:refnum<class "CoriFlowBFS1Plus.lvclass">)  [unwired: 16 in, 1 out]
        n160 = call-dynamic "ReadFlushBuffer.vi"("object in"=w403, "error in (no error)"=w401) -> ("object out"=w402:refnum<class "CoriFlowBFS1Plus.lvclass">, "Buffer"=→"Buffer":T13, "error out"=w400:errorcluster)  [unwired: 15 in]
        n161 = call-dynamic "SetCoriFlowBFS1Plus.vi"("object in"=w405, "CoriFlowBFS1Plus"=w402) -> ("object out"=w404:refnum<class "Application.lvclass">)  [unwired: 16 in, 1 out]
        n162 = Merge Errors(w400) -> (w407:errorcluster)
      }
      frame "ExperimentStart" {
        n163 = call-dynamic "FlushQueueMain.vi"("object in"=w411, "error in (no error)"=w408) -> ("object out"=w410:refnum<class "Application.lvclass">, "error out"=w409:errorcluster)  [unwired: 15 in, 1 out]
        n164 = call-dynamic "EnqueueMain.vi"("object in"=w410, "Message"="ExperimentRun") -> ("object out"=w412:refnum<class "Application.lvclass">)  [unwired: 16 in, 1 out]
      }
      frame "CoriolisFlushBuffer" {
        # "Duplicate this frame when creating new messages.  Change this comment in the duplicated frame to describe this message."
        n165 = call-dynamic "GetCoriFlowBFS1Plus.vi"("object in"=w422) -> ("object out"=w421:refnum<class "Application.lvclass">, "CoriFlowBFS1Plus"=w416:refnum<class "CoriFlowBFS1Plus.lvclass">)  [unwired: 16 in, 1 out]
        n166 = call-dynamic "ReadFlushBuffer.vi"("object in"=w416, "error in (no error)"=w417) -> ("object out"=w415:refnum<class "CoriFlowBFS1Plus.lvclass">, "error out"=w414:errorcluster)  [unwired: 15 in, 1 out]
        n167 = call-dynamic "SetCoriFlowBFS1Plus.vi"("object in"=w421, "CoriFlowBFS1Plus"=w415) -> ("object out"=w420:refnum<class "Application.lvclass">)  [unwired: 16 in, 1 out]
        n168 = call-dynamic "FireUpdateStatus.vi"("object in"=w420, "Status"="Coriolis Buffer Flushed") -> ("object out"=w419:refnum<class "Application.lvclass">)  [unwired: 16 in, 1 out]
        n169 = Merge Errors(w414) -> (w423:errorcluster)
      }
      frame "Error" {
        # "#CodeRecommended - If you ever change the name of this \"Error\" message, you'll need to update the name in the Check Loop Error.vi as well."
        # "#CodeRecommended - Consider creating a system for logging errors in some way. These errors are for notification purposes only. Handling of specific errors should be performed in the message frames that generated the error."
        # "Error - Display an error dialog. This message is sent by the \"Error Handler\" VIs at the end of other loops in this application."
        n170 = Variant To Data(error in=w430, type=errorcluster {"status"=FALSE, "code"=0, "source"=""} ("error constant"), Variant=w429) -> (data=w427:errorcluster, error out=w426:errorcluster)
        n171 = call <vilib>:"Simple Error Handler.vi"("error in (no error)"=w427) -> ()  [unwired: 4 in, 5 out]
        n172 = Merge Errors(w426) -> (w425:errorcluster)
      }
      frame "Exit" {
        # "Stop the VI"
        # "Release the message queue reference"
        # "#CodeNeeded - Add any required cleanup code here. Note that if 'Exit' was called as a result of an error, an error dialog will be displayed. Add any custom error handling for an 'Exit' condition here as well."
        # "Exit - Exit the application."
        n173 = call <vilib>:"Simple Error Handler.vi"("error in (no error)"=w432) -> ("error out"=w431:errorcluster)  [unwired: 4 in, 4 out]
        n174 = call-dynamic "FireStopEvent.vi"("object in"=w434, "error in (no error)"=w431) -> ("object out"=w435:refnum<class "Application.lvclass">, "error out"=w433:errorcluster)  [unwired: 16 in]
      }
      frame "ExperimentComplete" {
        # "Something - Replace this message with functionality for your own application."
        n175 = call-dynamic "GetExperiment.vi"("object in"=w447) -> ("object out"=w444:refnum<class "Application.lvclass">, "Experiment"=w441:refnum<class "Experiment.lvclass">)  [unwired: 16 in, 1 out]
        n176 = call-dynamic "CleanUp.vi"("object in"=w441, "error in (no error)"=w439) -> ("object out"=w442:refnum<class "Experiment.lvclass">, "error out"=w440:errorcluster)  [unwired: 16 in]
        n177 = call-dynamic "SetExperiment.vi"("object in"=w444, "Experiment"=w442) -> ("object out"=w443:refnum<class "Application.lvclass">)  [unwired: 16 in, 1 out]
        n178 = property on="Go Live" class="Bool (strict)"("DisabledEnum"=T16."Enabled" ("Disabled")) -> ()  [unwired: 2 in, 2 out]
        n179 = property on="Run Experiment" class="Bool"("DisabledEnum"=T16."Disabled" ("Disabled")) -> ()  [unwired: 2 in, 2 out]
        n180 = call-dynamic "FireUpdateStatus.vi"("object in"=w443, "Status"=" Experiment Complete....") -> ("object out"=w446:refnum<class "Application.lvclass">)  [unwired: 16 in, 1 out]
        n181 = Merge Errors(w440) -> (w448:errorcluster)
      }
      frame "ExperimentCreate" {
        # "Duplicate this frame when creating new messages.  Change this comment in the duplicated frame to describe this message."
        n182 = Variant To Data(error in=w466, type=path "" ("Experiment Base path"), Variant=w468) -> (data=w464:path, error out=w467:errorcluster)
        n183 = call "Experiment_Init.vi"("object in"=refnum<class "Experiment.lvclass"> refnum, "Path"=w464, "error in (no error)"=w467) -> ("object out"=w462:refnum<class "Experiment.lvclass">, "file or folder exists?"=w452:bool, "error out"=w460:errorcluster)  [unwired: 14 in]
        n184 = case shown="True" w452 {
          tunnel: w462 -> [w473 w482]
          tunnel: [w473 w481] -> w461
          tunnel: w460 -> [w472 w480]
          tunnel: [w472 w479] -> w459
          tunnel: "Number of Images at each Level" -> [_ w478]
          tunnel: "Ramp In (Experiment)" -> [_ w477]
          tunnel: "Levels (uL)" -> [_ w476]
          tunnel: "Triggering for experiment" -> [_ w475]
          tunnel: ["Experiment not created!!!" ("Status") "Experiment Created" ("Status")] -> w454
          frame False {
          }
          frame True {
            n185 = call-dynamic "Build Experiment.vi"("object in"=w482, "Triggering"=w475, "Levels"=w476, "Ramp In Settings"=w477, "Number of Images at each Level"=w478, "error in (no error)"=w480) -> ("object out"=w481:refnum<class "Experiment.lvclass">, "error out"=w479:errorcluster)  [unwired: 12 in]
          }
        }
        n186 = Select(t=T16."Enabled" ("Disabled"), s=w452, f=T16."Disabled and Grayed Out" ("Disabled")) -> (s? t:f=w450:T16)
        n187 = property on="Run Experiment" class="Bool"("DisabledEnum"=w450) -> ()  [unwired: 2 in, 2 out]
        n188 = call-dynamic "SetExperiment.vi"("object in"=w470, "Experiment"=w461) -> ("object out"=w469:refnum<class "Application.lvclass">)  [unwired: 16 in, 1 out]
        n189 = call-dynamic "FireUpdateStatus.vi"("object in"=w469, "Status"=w454) -> ("object out"=w455:refnum<class "Application.lvclass">)  [unwired: 16 in, 1 out]
      }
      frame "OpenImagePairWindows" {
        n190 = call-dynamic "GetHamamatsu.vi"("object in"=w492) -> ("object out"=w493:refnum<class "Application.lvclass">, "Hamamatsu"=w487:refnum<class "Hamamatsu.lvclass">)  [unwired: 16 in, 1 out]
        n191 = call-dynamic "GetImages.vi"("object in"=w487) -> ("object out"=w485:refnum<class "Hamamatsu.lvclass">, "HWSyncedImages"=w484:T22[])  [unwired: 16 in, 1 out]
        n192 = Build Array("Frame1" ("Title"), "Frame2" ("Title")) -> (w488:string[])
        n193 = call-dynamic "StoeDisplayImagesReference.vi"("object in"=w485, "Image Src"=w484) -> ("Images for Display Purpose"=w483:T22[])  [unwired: 15 in, 2 out]
        n194 = for {
          N: 2 -> [_]
          tunnel: w483 -> [w502] mode=indexing
          tunnel: w491 -> [w498]
          tunnel: w488 -> [w501] mode=indexing
          i -> [w500]
          n195 = Increment(x=w500) -> (x+1=w495:i32)
          n196 = call "IMAQ WindDraw"("Window Number (0...15)"=w495, "error in (no error)"=w498, "Title"=w501, "Image"=w502) -> ("error out"=w497:errorcluster)  [unwired: 6 in, 1 out]
          n197 = call "IMAQ WindShow"("error in (no error)"=w497, "Bring To Front? (N)"=TRUE, "Window Number (0...15)"=w495) -> ("error out"=w496:errorcluster)  [unwired: 3 in, 2 out]
          n198 = call "IMAQ WindZoom 2"("Window Number (0...15)"=w495, "error in (no error)"=w496, "Zoom to Fit? (False)"=TRUE) -> ()  [unwired: 5 in, 4 out]
        }
      }
      frame "ExperimentRun" {
        # "Something - Replace this message with functionality for your own application."
        n199 = call-dynamic "GetExperiment.vi"("object in"=w516, "error in (no error)"=w507) -> ("object out"=w513:refnum<class "Application.lvclass">, "Experiment"=w512:refnum<class "Experiment.lvclass">, "error out"=w506:errorcluster)  [unwired: 15 in]
        n200 = call-dynamic "DequeueExperiment.vi"("object in"=w512, "error in (no error)"=w506) -> ("QueueEmpty?"=w504:bool, "Message"=w510:string, "Message Data"=w509:variant, "Wait Command"=w503:bool, "error out"=w505:errorcluster)  [unwired: 12 in, 1 out]
        n201 = case shown="False" w504 {
          tunnel: w513 -> [w521 w529]
          tunnel: [w520 w523] -> w511
          tunnel: w510 -> [_ w528]
          tunnel: w509 -> [_ w527]
          tunnel: [w519 w526] -> w508
          tunnel: w505 -> [w518 w525]
          tunnel: w503 -> [_ w522]
          frame True {
            n202 = call-dynamic "EnqueueMain.vi"("object in"=w521, "Message"="ExperimentComplete", "error in (no error)"=w518) -> ("object out"=w520:refnum<class "Application.lvclass">, "error out"=w519:errorcluster)  [unwired: 15 in]
          }
          frame False {
            n203 = call-dynamic "EnqueueMain.vi"("object in"=w529, "Message"=w528, "Message Data"=w527, "error in (no error)"=w525) -> ("object out"=w524:refnum<class "Application.lvclass">, "error out"=w526:errorcluster)  [unwired: 14 in]
            n204 = case shown="True" w522 {
              tunnel: w524 -> [w532 w533]
              tunnel: [w531 w533] -> w523
              frame False {
                n205 = call-dynamic "EnqueueMain.vi"("object in"=w532, "Message"="ExperimentRun") -> ("object out"=w531:refnum<class "Application.lvclass">)  [unwired: 16 in, 1 out]
              }
              frame True {
              }
            }
          }
        }
        n206 = call-dynamic "FireUpdateStatus.vi"("object in"=w511, "Status"="Running Experiment....") -> ("object out"=w515:refnum<class "Application.lvclass">)  [unwired: 16 in, 1 out]
      }
      frame "HamamatsuCenterROI" {
        # "Duplicate this frame when creating new messages.  Change this comment in the duplicated frame to describe this message."
        n207 = call-dynamic "GetHamamatsu.vi"("object in"=w553, "error in (no error)"=w548) -> ("object out"=w552:refnum<class "Application.lvclass">, "Hamamatsu"=w550:refnum<class "Hamamatsu.lvclass">, "error out"=w537:errorcluster)  [unwired: 15 in]
        n208 = call-dynamic "StopCapture.vi"("object in"=w550, "error in (no error)"=w537) -> ("object out"=w538:refnum<class "Hamamatsu.lvclass">, "error out"=w536:errorcluster)  [unwired: 16 in]
        n209 = call-dynamic "CenterROI.vi"("object in"=w538, "error in (no error)"=w536) -> ("object out"=w549:refnum<class "Hamamatsu.lvclass">, "Sub Region"=w543:T24, "error out"=w547:errorcluster)  [unwired: 15 in]
        n210 = call-dynamic "SetHamamatsu.vi"("object in"=w552, "Hamamatsu"=w549, "error in (no error)"=w547) -> ("object out"=w551:refnum<class "Application.lvclass">, "error out"=w546:errorcluster)  [unwired: 15 in]
        n211 = Unbundle By Name(w543) -> ("H Offset.Value"=w542:i32, "V Offset.Value"=w541:i32, "H Size.Value"=w540:i32, "V Size.Value"=w539:i32)
        n212 = Bundle By Name(cluster=T10 {"Horizontal Offset"=0, "Vertical Offset"=0, "Horizontal Size"=0, "Vertical Size"=0} ("Sub Region"), "Horizontal Offset"=w542, "Vertical Offset"=w541, "Horizontal Size"=w540, "Vertical Size"=w539) -> (w544:T10)
        n213 = call-dynamic "FireUpdateStatus.vi"("object in"=w551, "Status"="ROI Centered") -> ("object out"=w535:refnum<class "Application.lvclass">)  [unwired: 16 in, 1 out]
        n214 = local write "ROI"(w544) -> ()
        n215 = Merge Errors(w546) -> (w554:errorcluster)
      }
      frame "HamamatsuConfigureROI" {
        # "Duplicate this frame when creating new messages.  Change this comment in the duplicated frame to describe this message."
        n216 = call-dynamic "GetHamamatsu.vi"("object in"=w574, "error in (no error)"=w571) -> ("object out"=w573:refnum<class "Application.lvclass">, "Hamamatsu"=w569:refnum<class "Hamamatsu.lvclass">, "error out"=w558:errorcluster)  [unwired: 15 in]
        n217 = call-dynamic "StopCapture.vi"("object in"=w569, "error in (no error)"=w558) -> ("object out"=w559:refnum<class "Hamamatsu.lvclass">, "error out"=w557:errorcluster)  [unwired: 16 in]
        n218 = call-dynamic "ConfigureROI.vi"("object in"=w559, "Sub Region"="ROI", "error in (no error)"=w557) -> ("object out"=w568:refnum<class "Hamamatsu.lvclass">, "SubRegionLimits"=w566:T25, "error out"=w567:errorcluster)  [unwired: 14 in]
        n219 = call-dynamic "SetHamamatsu.vi"("object in"=w573, "Hamamatsu"=w568, "error in (no error)"=w567) -> ("object out"=w572:refnum<class "Application.lvclass">, "error out"=w570:errorcluster)  [unwired: 15 in]
        n220 = Unbundle By Name(w566) -> ("H Offset.Value"=w563:i32, "V Offset.Value"=w562:i32, "H Size.Value"=w561:i32, "V Size.Value"=w560:i32)
        n221 = Merge Errors(w570) -> (w575:errorcluster)
        n222 = Bundle By Name(cluster="ROI", "Horizontal Offset"=w563, "Vertical Offset"=w562, "Horizontal Size"=w561, "Vertical Size"=w560) -> (w564:T10)
        n223 = call-dynamic "FireUpdateStatus.vi"("object in"=w572, "Status"="ROI Configured") -> ("object out"=w556:refnum<class "Application.lvclass">)  [unwired: 16 in, 1 out]
        n224 = local write "ROI"(w564) -> ()
      }
      frame "HamamatsuGetReadoutTime" {
        # "Duplicate this frame when creating new messages.  Change this comment in the duplicated frame to describe this message."
        n225 = call-dynamic "GetHamamatsu.vi"("object in"=w587, "error in (no error)"=w584) -> ("object out"=w586:refnum<class "Application.lvclass">, "Hamamatsu"=w582:refnum<class "Hamamatsu.lvclass">, "error out"=w580:errorcluster)  [unwired: 15 in]
        n226 = call-dynamic "ReadReadoutTime.vi"("object in"=w582, "error in (no error)"=w580) -> ("object out"=w581:refnum<class "Hamamatsu.lvclass">, "ReadoutTime"=→"ReadoutTime":dbl, "error out"=w579:errorcluster)  [unwired: 15 in]
        n227 = call-dynamic "SetHamamatsu.vi"("object in"=w586, "Hamamatsu"=w581, "error in (no error)"=w579) -> ("object out"=w585:refnum<class "Application.lvclass">, "error out"=w583:errorcluster)  [unwired: 15 in]
        n228 = call-dynamic "FireUpdateStatus.vi"("object in"=w585, "Status"="ReadOut Time aquired") -> ("object out"=w577:refnum<class "Application.lvclass">)  [unwired: 16 in, 1 out]
      }
      frame "HamamatsuGrabLive" {
        # "Duplicate this frame when creating new messages.  Change this comment in the duplicated frame to describe this message."
        n229 = call-dynamic "GetHamamatsu.vi"("object in"=w617, "error in (no error)"=w616) -> ("object out"=w605:refnum<class "Application.lvclass">, "Hamamatsu"=w614:refnum<class "Hamamatsu.lvclass">, "error out"=w606:errorcluster)  [unwired: 15 in]
        n230 = call-dynamic "GetAquisitionInProgress.vi"("object in"=w614, "error in (no error)"=w606) -> ("object out"=w602:refnum<class "Hamamatsu.lvclass">, "AquisitionInProgress?"=w596:bool, "AquisitionType"=w600:enum16{"HWSynced", "FreeRunning"}, "error out"=w603:errorcluster)  [unwired: 14 in]
        n231 = Not(x=w596) -> (.not. x?=w595:bool)
        n232 = Not Equal?(x=w600, y=enum16{"HWSynced", "FreeRunning"}."FreeRunning") -> (x != y?=w597:bool)
        n233 = Or(x=w595, y=w597) -> (x .or. y?=w598:bool)
        n234 = case shown="True" w598 {
          tunnel: [w618 w626] -> w604
          tunnel: w603 -> [w618 w625]
          tunnel: w602 -> [w619 w623]
          tunnel: [w619 w620] -> w601
          frame False {
          }
          frame True {
            n235 = call-dynamic "StopCapture.vi"("object in"=w623, "error in (no error)"=w625) -> ("object out"=w622:refnum<class "Hamamatsu.lvclass">, "error out"=w624:errorcluster)  [unwired: 16 in]
            n236 = call-dynamic "ConfigureFreeRunning.vi"("object in"=w622, "error in (no error)"=w624) -> ("object out"=w621:refnum<class "Hamamatsu.lvclass">, "error out"=w627:errorcluster)  [unwired: 16 in]
            n237 = call-dynamic "StartCapture.vi"("object in"=w621, "error in (no error)"=w627) -> ("object out"=w620:refnum<class "Hamamatsu.lvclass">, "error out"=w626:errorcluster)  [unwired: 16 in]
          }
        }
        n238 = call-dynamic "CaptureSnapshot.vi"("object in"=w601, "error in (no error)"=w604) -> ("object out"=w593:refnum<class "Hamamatsu.lvclass">, "FreeRunningImage"=w591:T22, "error out"=w589:errorcluster)  [unwired: 14 in, 1 out]
        n239 = local read "Go Live"() -> (w594:bool)
        n240 = call-dynamic "StoreDisplayImageReference.vi"("object in"=w593, "Image Src"=w591, "error in (no error)"=w589) -> ("object out"=w592:refnum<class "Hamamatsu.lvclass">, "Image Dst Out"=w590:T22, "error out"=w588:errorcluster)  [unwired: 14 in]
        n241 = call-dynamic "FireMessageEvent.vi"("object in"=w605, "Message"="UpdateLive", "Message Data"=w590) -> ("object out"=w612:refnum<class "Application.lvclass">)  [unwired: 15 in, 1 out]
        n242 = case shown="True" w594 {
          tunnel: [w629 w636] -> w615
          tunnel: w588 -> [w628 w635]
          tunnel: [w628 w634] -> w609
          tunnel: "HamamatsuGrabLive" ("Message") -> [_ w633]
          tunnel: w612 -> [w629 w632]
          tunnel: w592 -> [w630 w631]
          tunnel: [w630 w631] -> w610
          frame False {
          }
          frame True {
            n243 = call-dynamic "EnqueueMain.vi"("object in"=w632, "Message"=w633, "error in (no error)"=w635) -> ("object out"=w636:refnum<class "Application.lvclass">, "error out"=w634:errorcluster)  [unwired: 15 in]
          }
        }
        n244 = call-dynamic "SetHamamatsu.vi"("object in"=w615, "Hamamatsu"=w610, "error in (no error)"=w609) -> ("object out"=w611:refnum<class "Application.lvclass">, "error out"=w608:errorcluster)  [unwired: 15 in]
      }
      frame "HamamatsuInit" {
        # "Duplicate this frame when creating new messages.  Change this comment in the duplicated frame to describe this message."
        n245 = call-dynamic "FireUpdateStatus.vi"("object in"=w638, "Status"=w637) -> ("object out"=w639:refnum<class "Application.lvclass">)  [unwired: 16 in, 1 out]
        n246 = call-dynamic "GetHamamatsu.vi"("object in"=w639, "error in (no error)"=w653) -> ("object out"=w655:refnum<class "Application.lvclass">, "Hamamatsu"=w651:refnum<class "Hamamatsu.lvclass">, "error out"=w650:errorcluster)  [unwired: 15 in]
        n247 = call "Hamamatsu_Init.vi"("object in"=w651, "error in (no error)"=w650) -> ("object out"=w649:refnum<class "Hamamatsu.lvclass">, "error out"=w648:errorcluster)  [unwired: 16 in]
        n248 = call-dynamic "OpenCamera.vi"("object in"=w649, "error in (no error)"=w648) -> ("object out"=w645:refnum<class "Hamamatsu.lvclass">, "error out"=w643:errorcluster)  [unwired: 14 in, 2 out]
        n249 = control-ref of="ROI"() -> (w647:refnum<vi>)
        n250 = call-dynamic "ReadSubregionLimitsandValue.vi"("object in"=w645, "error in (no error)"=w643) -> ("object out"=w644:refnum<class "Hamamatsu.lvclass">, "Sub Region"=w641:T24, "error out"=w642:errorcluster)  [unwired: 15 in]
        n251 = call-dynamic "UpdateRoiLimits.vi"("object in"=w644, "reference to front panel item"=w647, "SubRegionLimits"=w641, "error in (no error)"=w642) -> ("object out"=w646:refnum<class "Hamamatsu.lvclass">, "error out"=w640:errorcluster)  [unwired: 14 in]
        n252 = call-dynamic "SetHamamatsu.vi"("object in"=w655, "Hamamatsu"=w646, "error in (no error)"=w640) -> ("object out"=w654:refnum<class "Application.lvclass">, "error out"=w652:errorcluster)  [unwired: 15 in]
      }
      frame "HamamatsuSetExposureTime" {
        # "Duplicate this frame when creating new messages.  Change this comment in the duplicated frame to describe this message."
        n253 = call-dynamic "GetHamamatsu.vi"("object in"=w665, "error in (no error)"=w662) -> ("object out"=w664:refnum<class "Application.lvclass">, "Hamamatsu"=w660:refnum<class "Hamamatsu.lvclass">, "error out"=w658:errorcluster)  [unwired: 15 in]
        n254 = call-dynamic "ConfigureExposureTime.vi"("object in"=w660, "ExposureTime(ms)"="Exposure (ms)", "error in (no error)"=w658) -> ("object out"=w659:refnum<class "Hamamatsu.lvclass">, "error out"=w657:errorcluster)  [unwired: 15 in]
        n255 = call-dynamic "SetHamamatsu.vi"("object in"=w664, "Hamamatsu"=w659, "error in (no error)"=w657) -> ("object out"=w663:refnum<class "Application.lvclass">, "error out"=w661:errorcluster)  [unwired: 15 in]
      }
      frame "HamamatsuStartHWTimedAquisition" {
        n256 = call-dynamic "GetHamamatsu.vi"("object in"=w680, "error in (no error)"=w676) -> ("object out"=w679:refnum<class "Application.lvclass">, "Hamamatsu"=w669:refnum<class "Hamamatsu.lvclass">, "error out"=w667:errorcluster)  [unwired: 15 in]
        n257 = call-dynamic "StopCapture.vi"("object in"=w669, "error in (no error)"=w667) -> ("object out"=w668:refnum<class "Hamamatsu.lvclass">, "error out"=w666:errorcluster)  [unwired: 16 in]
        n258 = call-dynamic "ConfigureHWSynced.vi"("object in"=w668, "FramesPerAquisionCycle"=2, "CameraBufferSize"=10, "error in (no error)"=w666) -> ("object out"=w673:refnum<class "Hamamatsu.lvclass">, "error out"=w671:errorcluster)  [unwired: 14 in]
        n259 = call-dynamic "StartCapture.vi"("object in"=w673, "error in (no error)"=w671) -> ("object out"=w672:refnum<class "Hamamatsu.lvclass">, "error out"=w670:errorcluster)  [unwired: 16 in]
        n260 = call-dynamic "SetHamamatsu.vi"("object in"=w679, "Hamamatsu"=w672, "error in (no error)"=w670) -> ("object out"=w675:refnum<class "Application.lvclass">, "error out"=w674:errorcluster)  [unwired: 15 in]
      }
      frame "HamamatsuStartLive" {
        # "Duplicate this frame when creating new messages.  Change this comment in the duplicated frame to describe this message."
        n261 = call-dynamic "GetHamamatsu.vi"("object in"=w696, "error in (no error)"=w693) -> ("object out"=w695:refnum<class "Application.lvclass">, "Hamamatsu"=w692:refnum<class "Hamamatsu.lvclass">, "error out"=w682:errorcluster)  [unwired: 15 in]
        n262 = call-dynamic "StopCapture.vi"("object in"=w692, "error in (no error)"=w682) -> ("object out"=w683:refnum<class "Hamamatsu.lvclass">, "error out"=w681:errorcluster)  [unwired: 16 in]
        n263 = call-dynamic "ConfigureFreeRunning.vi"("object in"=w683, "error in (no error)"=w681) -> ("object out"=w691:refnum<class "Hamamatsu.lvclass">, "error out"=w689:errorcluster)  [unwired: 16 in]
        n264 = call-dynamic "StartCapture.vi"("object in"=w691, "error in (no error)"=w689) -> ("object out"=w690:refnum<class "Hamamatsu.lvclass">, "error out"=w688:errorcluster)  [unwired: 16 in]
        n265 = call-dynamic "SetHamamatsu.vi"("object in"=w695, "Hamamatsu"=w690, "error in (no error)"=w688) -> ("object out"=w694:refnum<class "Application.lvclass">, "error out"=w685:errorcluster)  [unwired: 15 in]
        n266 = call-dynamic "EnqueueMain.vi"("object in"=w694, "Message"="HamamatsuGrabLive", "error in (no error)"=w685) -> ("object out"=w687:refnum<class "Application.lvclass">, "error out"=w686:errorcluster)  [unwired: 15 in]
      }
      frame "HamamatsuStopCapture" {
        # "Duplicate this frame when creating new messages.  Change this comment in the duplicated frame to describe this message."
        n267 = call-dynamic "GetHamamatsu.vi"("object in"=w705, "error in (no error)"=w704) -> ("object out"=w701:refnum<class "Application.lvclass">, "Hamamatsu"=w700:refnum<class "Hamamatsu.lvclass">, "error out"=w699:errorcluster)  [unwired: 15 in]
        n268 = call-dynamic "StopCapture.vi"("object in"=w700, "error in (no error)"=w699) -> ("object out"=w698:refnum<class "Hamamatsu.lvclass">, "error out"=w697:errorcluster)  [unwired: 16 in]
        n269 = call-dynamic "SetHamamatsu.vi"("object in"=w701, "Hamamatsu"=w698, "error in (no error)"=w697) -> ("object out"=w703:refnum<class "Application.lvclass">, "error out"=w702:errorcluster)  [unwired: 15 in]
      }
      frame "HamamatsuCaptureHWtimedImages" {
        n270 = call-dynamic "GetAD2_SDK.vi"("object in"=w727) -> ("object out"=w728:refnum<class "Application.lvclass">, "AD2_SDK"=w729:refnum<class "AD2_SDK.lvclass">)  [unwired: 16 in, 1 out]
        n271 = call-dynamic "PCTrig.vi"("object in"=w729, "error in (no error)"=w731) -> ("object out"=w730:refnum<class "AD2_SDK.lvclass">, "error out"=w726:errorcluster)  [unwired: 16 in]
        n272 = call-dynamic "SetAD2_SDK.vi"("object in"=w728, "AD2_SDK"=w730) -> ("object out"=w723:refnum<class "Application.lvclass">)  [unwired: 16 in, 1 out]
        n273 = call-dynamic "FireUpdateStatus.vi"("object in"=w723, "Status"="Waiting for HW timed images") -> ("object out"=w722:refnum<class "Application.lvclass">)  [unwired: 16 in, 1 out]
        n274 = call-dynamic "GetHamamatsu.vi"("object in"=w722, "error in (no error)"=w726) -> ("object out"=w721:refnum<class "Application.lvclass">, "Hamamatsu"=w736:refnum<class "Hamamatsu.lvclass">, "error out"=w735:errorcluster)  [unwired: 15 in]
        n275 = while {
          shift-right: [w749] -> w733
          shift-left: w736 -> [w751]
          shift-right: [w748] -> w717
          shift-left: w735 -> [w750]
          tunnel: w721 -> [w747]
          tunnel: [w746] -> w720
          tunnel: [w741] -> w714
          shift-right: [w741] -> _
          shift-left: TRUE ("Time has Elapsed") -> [w740]
          stop <- w742 stop-if-true
          n276 = call-dynamic "PreviewQueueMain.vi"("object in"=w747, "timeout in ms (-1)"=0) -> ("object out"=w746:refnum<class "Application.lvclass">, "Message"=w745:string)  [unwired: 14 in, 2 out]
          n277 = call "Elapsed Time"("Time Target (s)"=10.0, "Reset"=w740) -> ("Time has Elapsed"=w741:bool)  [unwired: 10 in, 7 out]
          n278 = call-dynamic "CaptureHWSynced.vi"("object in"=w751, "error in (no error)"=w750) -> ("object out"=w749:refnum<class "Hamamatsu.lvclass">, "AllFramesAvailable?"=w743:bool, "error out"=w748:errorcluster)  [unwired: 13 in, 2 out]
          n279 = case shown="\"False\", Default" w745 {
            tunnel: [_ TRUE] -> w744
            frame "False", Default {
            }
            frame "Abort", "Error", "Exit" {
            }
          }
          n280 = Compound Arithmetic op=OR(w744, w743, w741) -> (w742:bool)
        }
        n281 = call-dynamic "GetImages.vi"("object in"=w733, "error in (no error)"=w717) -> ("object out"=w709:refnum<class "Hamamatsu.lvclass">, "HWSyncedImages"=w711:T22[], "error out"=w707:errorcluster)  [unwired: 15 in]
        n282 = call-dynamic "StoeDisplayImagesReference.vi"("object in"=w709, "Image Src"=w711, "error in (no error)"=w707) -> ("object out"=w708:refnum<class "Hamamatsu.lvclass">, "Images for Display Purpose"=w710:T22[], "error out"=w706:errorcluster)  [unwired: 14 in]
        n283 = call-dynamic "SetHamamatsu.vi"("object in"=w720, "Hamamatsu"=w708, "error in (no error)"=w706) -> ("object out"=w732:refnum<class "Application.lvclass">, "error out"=w718:errorcluster)  [unwired: 15 in]
        n284 = call-dynamic "FireMessageEvent.vi"("object in"=w732, "Message"="UpdateHWTimed", "Message Data"=w710, "error in (no error)"=w718) -> ("object out"=w725:refnum<class "Application.lvclass">, "error out"=w734:errorcluster)  [unwired: 14 in]
        n285 = Select(t="Timout Occured Check DIO Settings", s=w714, f="HW Images Aquired" ("Status")) -> (s? t:f=w715:string)
        n286 = call-dynamic "FireUpdateStatus.vi"("object in"=w725, "Status"=w715) -> ("object out"=w737:refnum<class "Application.lvclass">)  [unwired: 16 in, 1 out]
      }
      frame "Initialize" {
        # "Initialize - All initialization work should take place in this message, since other loops can potentially enqueue messages that execute immediately after this one."
        n287 = Build Array("CoriolisInit", "CetoniInit", "HamamatsuInit", "AD2Init") -> (w758:string[])
        n288 = for {
          shift-right: [w762] -> w756
          shift-left: w755 -> [w763]
          tunnel: w758 -> [w761] mode=indexing
          n289 = call-dynamic "EnqueueMain.vi"("object in"=w763, "Message"=w761) -> ("object out"=w762:refnum<class "Application.lvclass">)  [unwired: 16 in, 1 out]
        }
      }
      frame "InjectError" {
        # "Something Else - Replace this message with functionality for your own application."
        n290 = Variant To Data(error in=w765, type=errorcluster {"status"=FALSE, "code"=0, "source"=""} ("error in (no error)"), Variant=w768) -> (data=w764:errorcluster, error out=w766:errorcluster)
        n291 = Merge Errors(w764, w766) -> (w770:errorcluster)
      }
      frame "ReadAndSaveData" {
        # "Duplicate this frame when creating new messages.  Change this comment in the duplicated frame to describe this message."
        n292 = call-dynamic "GetCoriFlowBFS1Plus.vi"("object in"=w784) -> ("object out"=w783:refnum<class "Application.lvclass">, "CoriFlowBFS1Plus"=w774:refnum<class "CoriFlowBFS1Plus.lvclass">)  [unwired: 16 in, 1 out]
        n293 = call-dynamic "ReadLatest.vi"("object in"=w774, "error in (no error)"=w776) -> ("object out"=w773:refnum<class "CoriFlowBFS1Plus.lvclass">, "Latest Data"=w775:T14, "error out"=w772:errorcluster)  [unwired: 15 in]
        n294 = Unbundle By Name(w775) -> ("Cluster"=w771:T12)
        n295 = call-dynamic "ReadFlushBuffer.vi"("object in"=w773, "error in (no error)"=w772) -> ("Buffer"=w777:T13, "error out"=w778:errorcluster)  [unwired: 15 in, 1 out]
        n296 = call-dynamic "FireMessageEvent.vi"("object in"=w783, "Message"="UpdateCoriolis", "Message Data"=w771) -> ("object out"=w782:refnum<class "Application.lvclass">)  [unwired: 15 in, 1 out]
        n297 = call-dynamic "GetHamamatsu.vi"("object in"=w782, "error in (no error)"=w778) -> ("object out"=w789:refnum<class "Application.lvclass">, "Hamamatsu"=w804:refnum<class "Hamamatsu.lvclass">, "error out"=w800:errorcluster)  [unwired: 15 in]
        n298 = call-dynamic "GetImages.vi"("object in"=w804, "error in (no error)"=w800) -> ("object out"=w796:refnum<class "Hamamatsu.lvclass">, "HWSyncedImages"=w799:T22[], "error out"=w795:errorcluster)  [unwired: 15 in]
        n299 = call-dynamic "GetArrayOfTimestamps.vi"("object in"=w796, "error in (no error)"=w795) -> ("Array of timestamps"=w792:dbl[], "error out"=w780:errorcluster)  [unwired: 15 in, 1 out]
        n300 = call-dynamic "GetCetoniPump.vi"("object in"=w789) -> ("object out"=w787:refnum<class "Application.lvclass">, "CetoniPump"=w786:refnum<class "CetoniPump.lvclass">)  [unwired: 16 in, 1 out]
        n301 = call-dynamic "ReadStatusAllPumps.vi"("object in"=w786, "error in (no error)"=w780) -> ("Array"=w785:T2, "error out"=w779:errorcluster)  [unwired: 15 in, 1 out]
        n302 = call-dynamic "GetExperiment.vi"("object in"=w787, "error in (no error)"=w779) -> ("object out"=w788:refnum<class "Application.lvclass">, "Experiment"=w803:refnum<class "Experiment.lvclass">, "error out"=w798:errorcluster)  [unwired: 15 in]
        n303 = call-dynamic "SaveImages.vi"("object in"=w803, "Images"=w799, "error in (no error)"=w798) -> ("object out"=w801:refnum<class "Experiment.lvclass">, "FileNames"=w793:string[], "error out"=w791:errorcluster)  [unwired: 14 in]
        n304 = call-dynamic "WriteTDMS.vi"("object in"=w801, "Pump Array"=w785, "FileNames"=w793, "Array of timestamps"=w792, "error in (no error)"=w791, "Coriols Async Data"=w777, "Coriolis Data"=w771) -> ("object out"=w794:refnum<class "Experiment.lvclass">, "error out"=w790:errorcluster)  [unwired: 11 in]
        n305 = call-dynamic "SetExperiment.vi"("object in"=w788, "Experiment"=w794, "error in (no error)"=w790) -> ("object out"=w802:refnum<class "Application.lvclass">, "error out"=w797:errorcluster)  [unwired: 15 in]
      }
      frame "SaveImages" {
        # "Duplicate this frame when creating new messages.  Change this comment in the duplicated frame to describe this message."
        n306 = call-dynamic "GetHamamatsu.vi"("object in"=w815, "error in (no error)"=w814) -> ("object out"=w811:refnum<class "Application.lvclass">, "Hamamatsu"=w810:refnum<class "Hamamatsu.lvclass">, "error out"=w808:errorcluster)  [unwired: 15 in]
        n307 = call-dynamic "GetImages.vi"("object in"=w810, "error in (no error)"=w808) -> ("object out"=w809:refnum<class "Hamamatsu.lvclass">, "HWSyncedImages"=w806:T22[], "error out"=w807:errorcluster)  [unwired: 15 in]
        n308 = call-dynamic "SetHamamatsu.vi"("object in"=w811, "Hamamatsu"=w809, "error in (no error)"=w807) -> ("object out"=w813:refnum<class "Application.lvclass">, "error out"=w812:errorcluster)  [unwired: 15 in]
        n309 = for {
          tunnel: w806 -> [w825] mode=indexing
          w823 = 5 ("Window Number (0...15)")
          n310 = call "IMAQ WindShow"("Bring To Front? (N)"=TRUE, "Window Number (0...15)"=w823) -> ("error out"=w821:errorcluster)  [unwired: 4 in, 2 out]
          n311 = call "IMAQ WindDraw"("Window Number (0...15)"=w823, "error in (no error)"=w821, "Title"="Image to save", "Image"=w825) -> ("error out"=w817:errorcluster)  [unwired: 6 in, 1 out]
          n312 = call "File Dialog"("start path"=path "c:/", "prompt"="Save Image(s)", "error in"=w817, "pattern (all files)"=".tif") -> ("selected path"=w826:path, "cancelled"=w818:bool, "error out"=w816:errorcluster)  [unwired: 8 in, 1 out]
          n313 = call <vilib>:"Clear Errors.vi"("error in (no error)"=w816) -> ()  [unwired: 5 in, 2 out]
          n314 = case shown="False" w818 {
            tunnel: w826 -> [w829 _]
            tunnel: w825 -> [w828 _]
            frame False {
              n315 = call-poly "IMAQ Write File 2"("File Path"=w829, "Image"=w828) -> ()  [unwired: 8 in, 2 out]
            }
            frame True {
            }
          }
        }
        n316 = call-dynamic "FireUpdateStatus.vi"("object in"=w813) -> ("object out"=w805:refnum<class "Application.lvclass">)  [unwired: 17 in, 1 out]
      }
      frame "Something" {
        # "Send string to \"Update Display\" message"
        # "#CodeNeeded - Perform whatever actions correspond to the \"Something\" message."
        # "Something - Replace this message with functionality for your own application."
        n317 = Merge Errors(w831) -> (w832:errorcluster)
      }
      frame "WaitTime" {
        n318 = local read "Wait"() -> (w833:T15)
        n319 = Variant To Data(error in=w843, type=w833, Variant=w844) -> (data=w842:T15)  [unwired: 1 out]
        n320 = Unbundle By Name(w842) -> ("Wait Time"=w835:dbl, "Reset"=w839:bool, "Part of Experiment"=w837:bool)
        n321 = call "Elapsed Time"("Time Target (s)"=w835, "Reset"=w839, "Auto Reset"=FALSE) -> ("Time has Elapsed"=w838:bool, "Elapsed Time Text"=w836:string)  [unwired: 9 in, 6 out]
        n322 = Bundle By Name(cluster=w842, "Reset"=FALSE) -> (w841:T15)
        n323 = case shown="True" w838 {
          tunnel: w846 -> [w858 w866]
          tunnel: [w854 w860] -> w845
          tunnel: w841 -> [w855 _]
          tunnel: w837 -> [_ w859]
          tunnel: w836 -> [w851 w862]
          tunnel: w835 -> [w850 _]
          frame False {
            n324 = Number To Fractional String(number=w850) -> (F-format string=w848:string)  [unwired: 3 in]
            n325 = call-dynamic "EnqueueMain.vi"("object in"=w858, "Message"="WaitTime", "Message Data"=w855) -> ("object out"=w857:refnum<class "Application.lvclass">)  [unwired: 15 in, 1 out]
            n326 = Concatenate Strings("Waiting " ("Status"), w851, "/" ("string"), w848, " s" ("string")) -> (w852:string)
            n327 = call-dynamic "FireUpdateStatus.vi"("object in"=w857, "Status"=w852) -> ("object out"=w854:refnum<class "Application.lvclass">)  [unwired: 16 in, 1 out]
          }
          frame True {
            n328 = Concatenate Strings("Wait Complete" ("Status"), w862, "s" ("string")) -> (w863:string)
            n329 = call-dynamic "FireUpdateStatus.vi"("object in"=w866, "Status"=w863) -> ("object out"=w865:refnum<class "Application.lvclass">)  [unwired: 16 in, 1 out]
            n330 = case shown="True" w859 {
              tunnel: w865 -> [w867 w870]
              tunnel: [w867 w869] -> w860
              frame False {
              }
              frame True {
                n331 = call-dynamic "EnqueueMain.vi"("object in"=w870, "Message"="ExperimentRun") -> ("object out"=w869:refnum<class "Application.lvclass">)  [unwired: 16 in, 1 out]
              }
            }
          }
        }
      }
      frame Default {
        # "'Default' case only runs if there is a message that isn't defined in any of the other cases.  Output a programming error."
        n332 = xnode "Error Ring"("parameter 0"=w872) -> ("error out"=w873:errorcluster)
      }
    }
    n333 = call-dynamic "ErrorHandlerMainLoop.vi"("object in"=w18, "error in (no error)"=w21) -> ("object out"=w19:refnum<class "Application.lvclass">, "error out"=w20:errorcluster)  [unwired: 16 in]
  }
  n334 = while {
    shift-right: [w888] -> _
    shift-left: w14 -> [w889]
    tunnel: [w883] -> w8
    shift-right: [w881] -> _
    shift-left: w13 -> [w886]
    tunnel: w12 -> [w885]
    stop <- w887 stop-if-true
    # "Event Handling Loop"
    n335 = event shown="[16] \"Open Live Window\": Value Change" {
      selector: w889 -> [_ _ _ _ _ _ _ _ _ _ _ _ _ _ _ _ _ _ _ _ _ _ _ _ _ _ _ _ _ _ _ _ _ _ _ _]
      dyn-events: [_ _ _ _ _ _ _ _ _ _ _ _ _ _ _ _ _ _ _ _ _ _ _ _ _ _ _ _ _ _ _ _ _ _ _ _] -> w888
      timeout: _ -> [_ _ _ _ _ _ _ _ _ _ _ _ _ _ _ _ _ _ _ _ _ _ _ _ _ _ _ _ _ _ _ _ _ _ _ _]
      tunnel: [_ _ _ _ _ _ _ _ _ _ _ _ _ _ _ _ _ _ _ _ _ _ _ _ _ _ _ _ _ _ _ _ _ TRUE ("Discard?") _ _] -> w887
      tunnel: [w891 w899 _ w906 _ _ _ _ w929 _ w936 w940 w945 w951 w958 w963 _ _ w982 w1001 w1004 w1009 w1014 _ _ w1029 _ w1039 w1045 w1051 w1056 w1058 w1066 w1072 w1078 _] -> w884
      tunnel: w886 -> [w894 w901 w905 w911 w915 w920 w923 w926 w932 w935 w939 w943 w948 w954 w961 w966 w977 w980 w985 w1002 w1007 w1012 w1021 w1024 w1027 w1032 w1036 w1042 w1048 w1050 w1057 w1063 w1071 w1075 w1081 w1156]
      tunnel: [w893 w895 w904 w910 w914 w921 w923 w925 w931 w934 w938 w942 w947 w953 w960 w965 w977 w979 w984 w1002 w1006 w1011 w1016 w1023 w1026 w1031 w1036 w1041 w1047 w1049 w1057 w1062 w1070 w1075 w1081 w1158] -> w882
      tunnel: w885 -> [w890 w898 _ w907 _ _ _ _ w928 _ w936 w940 w944 w950 w957 w962 _ _ w981 w1001 w1003 w1008 w1019 _ _ w1028 _ w1038 w1044 w1052 w1056 w1059 w1067 w1073 w1079 _]
      event "Save HW Timed Image Pair": Value Change {
        n336 = event-data() -> ()  [unwired: 1 in, 1 out]
        n337 = call-dynamic "EnqueueMain.vi"("object in"=w894, "Message"="SaveImages", "error in (no error)"=w890) -> ("object out"=w893:refnum<class "Application.lvclass">, "error out"=w891:errorcluster)  [unwired: 15 in]
      }
      event "Take HW Timed Image Pair": Value Change {
        n338 = event-data() -> ()  [unwired: 1 in, 1 out]
        n339 = call-dynamic "EnqueueMain.vi"("object in"=w901, "Message"="HamamatsuStartHWTimedAquisition", "error in (no error)"=w898) -> ("object out"=w896:refnum<class "Application.lvclass">, "error out"=w899:errorcluster)  [unwired: 15 in]
        n340 = call-dynamic "EnqueueMain.vi"("object in"=w896, "Message"="HamamatsuCaptureHWtimedImages") -> ("object out"=w895:refnum<class "Application.lvclass">)  [unwired: 16 in, 1 out]
      }
      event "Configure Triggering": Value Change {
        n341 = event-data() -> ()  [unwired: 1 in, 2 out]
        n342 = call-dynamic "EnqueueMain.vi"("object in"=w905, "Message"="AD2ConfigureDO", "Message Data"="Triggering") -> ("object out"=w904:refnum<class "Application.lvclass">)  [unwired: 15 in, 1 out]
      }
      event "Create Experiment": Value Change {
        n343 = event-data() -> ()  [unwired: 1 in, 2 out]
        n344 = call-dynamic "EnqueueMain.vi"("object in"=w911, "Message"="ExperimentCreate", "Message Data"="Experiment Base path", "error in (no error)"=w907) -> ("object out"=w910:refnum<class "Application.lvclass">, "error out"=w906:errorcluster)  [unwired: 14 in]
      }
      event "Wait": Value Change {
        n345 = event-data() -> ()  [unwired: 1 in, 2 out]
        n346 = call-dynamic "EnqueueMain.vi"("object in"=w915, "Message"="WaitTime", "Message Data"="Wait") -> ("object out"=w914:refnum<class "Application.lvclass">)  [unwired: 15 in, 1 out]
      }
      event "Ramp IN flow": Value Change {
        n347 = event-data() -> ()  [unwired: 1 in, 2 out]
        n348 = Bundle("Ramp In Settings"="Ramp In Settings", FALSE) -> (w916:T20)  [unwired: 1 in]
        n349 = call-dynamic "EnqueueMain.vi"("object in"=w920, "Message"="CetoniWaitRampIn", "Message Data"=w916) -> ("object out"=w921:refnum<class "Application.lvclass">)  [unwired: 15 in, 1 out]
      }
      event "Read Trigges Values From HW Timed TAB": Value Change {
        n350 = event-data() -> ()  [unwired: 1 in, 2 out]
        n351 = local read "Triggering"() -> (w922:T11)
        n352 = local write "Triggering for experiment"(w922) -> ()
      }
      event "Read Current Syringe \nConfiguration": Value Change {
        n353 = event-data() -> ()  [unwired: 1 in, 2 out]
        n354 = call-dynamic "EnqueueMain.vi"("object in"=w926, "Message"="CetoniReadCurrentSyringes") -> ("object out"=w925:refnum<class "Application.lvclass">)  [unwired: 16 in, 1 out]
      }
      event "Cetoni Wait for Level": Value Change {
        n355 = event-data() -> ()  [unwired: 1 in, 1 out]
        n356 = call-dynamic "EnqueueMain.vi"("object in"=w932, "Message"="CetoniWaitForLevel", "Message Data"="CetoniWaitData", "error in (no error)"=w928) -> ("object out"=w931:refnum<class "Application.lvclass">, "error out"=w929:errorcluster)  [unwired: 14 in]
      }
      event "Connect TO Hardware": Value Change {
        n357 = event-data() -> ()  [unwired: 1 in, 2 out]
        n358 = call-dynamic "EnqueueMain.vi"("object in"=w935, "Message"="Initialize") -> ("object out"=w934:refnum<class "Application.lvclass">)  [unwired: 16 in, 1 out]
      }
      event "Read Coriolis": Value Change {
        n359 = event-data() -> ()  [unwired: 1 in, 2 out]
        n360 = call-dynamic "EnqueueMain.vi"("object in"=w939, "Message"="CoriolisMeasure") -> ("object out"=w938:refnum<class "Application.lvclass">)  [unwired: 16 in, 1 out]
      }
      event "Read Coriolis Buffer": Value Change {
        n361 = event-data() -> ()  [unwired: 1 in, 2 out]
        n362 = call-dynamic "EnqueueMain.vi"("object in"=w943, "Message"="CoriolisReadBuffer") -> ("object out"=w942:refnum<class "Application.lvclass">)  [unwired: 16 in, 1 out]
      }
      event "Center ROI": Value Change {
        n363 = event-data() -> ()  [unwired: 1 in, 1 out]
        n364 = call-dynamic "EnqueueMain.vi"("object in"=w948, "Message"="HamamatsuCenterROI", "error in (no error)"=w944) -> ("object out"=w947:refnum<class "Application.lvclass">, "error out"=w945:errorcluster)  [unwired: 15 in]
      }
      event "Go Live": Value Change {
        n365 = event-data() -> ()  [unwired: 1 in, 1 out]
        n366 = call-dynamic "EnqueueMain.vi"("object in"=w954, "Message"="HamamatsuStartLive", "error in (no error)"=w950) -> ("object out"=w953:refnum<class "Application.lvclass">, "error out"=w951:errorcluster)  [unwired: 15 in]
        n367 = case shown="False" "Go Live" {
          frame False {
            n368 = property on="Take HW Timed Image Pair" class="Bool"("DisabledEnum"=T16."Enabled" ("Disabled")) -> ()  [unwired: 2 in, 2 out]
          }
          frame True {
            n369 = property on="Take HW Timed Image Pair" class="Bool"("DisabledEnum"=T16."Disabled and Grayed Out" ("Disabled")) -> ()  [unwired: 2 in, 2 out]
          }
        }
      }
      event "Configure ROI": Value Change {
        n370 = event-data() -> ()  [unwired: 1 in, 1 out]
        n371 = call-dynamic "EnqueueMain.vi"("object in"=w961, "Message"="HamamatsuConfigureROI", "error in (no error)"=w957) -> ("object out"=w960:refnum<class "Application.lvclass">, "error out"=w958:errorcluster)  [unwired: 15 in]
      }
      event "Read Redout Time": Value Change {
        n372 = event-data() -> ()  [unwired: 1 in, 1 out]
        n373 = call-dynamic "EnqueueMain.vi"("object in"=w966, "Message"="HamamatsuGetReadoutTime", "error in (no error)"=w962) -> ("object out"=w965:refnum<class "Application.lvclass">, "error out"=w963:errorcluster)  [unwired: 15 in]
      }
      event "Open Live Window": Value Change {
        w969 = 0 ("Window Number (0...15)")
        n374 = event-data() -> ()  [unwired: 1 in, 2 out]
        n375 = call "IMAQ Create"("Border Size"=3, "Image Name"="test image") -> ("New Image"=w973:T22)  [unwired: 3 in, 1 out]
        n376 = call "IMAQ WindShow"("Bring To Front? (N)"=TRUE, "Window Number (0...15)"=w969) -> ("error out"=w975:errorcluster)  [unwired: 4 in, 2 out]
        n377 = call "IMAQ WindDraw"("Resize to Image Size? (Y)"=FALSE, "Window Number (0...15)"=w969, "error in (no error)"=w975, "Title"="Live Image", "Image"=w973) -> ("error out"=w968:errorcluster)  [unwired: 5 in, 1 out]
        n378 = call "IMAQ WindZoom 2"("Window Number (0...15)"=w969, "error in (no error)"=w968, "Zoom to Fit? (False)"=TRUE) -> ()  [unwired: 5 in, 4 out]
      }
      event "Open Image Pairs Windows": Value Change {
        n379 = event-data() -> ()  [unwired: 1 in, 2 out]
        n380 = call-dynamic "EnqueueMain.vi"("object in"=w980, "Message"="OpenImagePairWindows") -> ("object out"=w979:refnum<class "Application.lvclass">)  [unwired: 16 in, 1 out]
      }
      event "Set Exposure Time": Value Change {
        n381 = event-data() -> ()  [unwired: 1 in, 1 out]
        n382 = call-dynamic "EnqueueMain.vi"("object in"=w985, "Message"="HamamatsuSetExposureTime", "error in (no error)"=w981) -> ("object out"=w984:refnum<class "Application.lvclass">, "error out"=w982:errorcluster)  [unwired: 15 in]
      }
      event "Open DIO signal helper": Value Change {
        n383 = event-data() -> ()  [unwired: 1 in, 2 out]
        n384 = Current VI's Path() -> (path=w992:path)
        n385 = Strip Path(path=w992) -> (stripped path=w995:path)  [unwired: 1 out]
        n386 = Build Path(base path=w995, name or relative path="VisualizeTriggerTiming.vi") -> (appended path=w993:path)
        n387 = Open VI Reference(type specifier VI Refnum (for type only)=refnum<vi> refnum, vi path=w993, options=128) -> (vi reference=w994:refnum<vi>)  [unwired: 3 in, 1 out]
        n388 = local read "Exposure (ms)"() -> (w999:dbl)
        n389 = local read "ReadoutTime"() -> (w1000:dbl)
        n390 = invoke class="VI (strict)" method="FP.Open"(reference=w994, "Activate"=TRUE ("Activate?"), "State"=T26."Standard") -> (reference out=w996:refnum<vi>)  [unwired: 2 in, 4 out]
        n391 = local read "Triggering"() -> (w987:T11)
        n392 = call-by-ref "Start Asynchronous Call"(reference=w996, "Pulse Settings"=w987, "Exposure Time (ms)"=w999, "ReadoutTime"=w1000) -> (reference out=w997:refnum<vi>, error out=w998:errorcluster)  [unwired: 17 in, 1 out]
        n393 = Close Reference(reference=w997, error in (no error)=w998) -> ()  [unwired: 1 out]
      }
      event "ReferenceMove": Value Change {
        n394 = event-data() -> ()  [unwired: 1 in, 1 out]
        n395 = call-dynamic "EnqueueMain.vi"("object in"=w1007, "Message"="CetoniReferenceMove", "error in (no error)"=w1003) -> ("object out"=w1006:refnum<class "Application.lvclass">, "error out"=w1004:errorcluster)  [unwired: 15 in]
      }
      event "ReadStatus": Value Change {
        n396 = event-data() -> ()  [unwired: 1 in, 1 out]
        n397 = call-dynamic "EnqueueMain.vi"("object in"=w1012, "Message"="CetoniReadStatus", "error in (no error)"=w1008) -> ("object out"=w1011:refnum<class "Application.lvclass">, "error out"=w1009:errorcluster)  [unwired: 15 in]
      }
      event "ConfigureSyringe": Value Change {
        n398 = event-data() -> ()  [unwired: 1 in, 1 out]
        n399 = call-dynamic "EnqueueMain.vi"("object in"=w1021, "Message"="CetoniConfigureSyringe", "Message Data"="SyringeSettings", "error in (no error)"=w1019) -> ("object out"=w1017:refnum<class "Application.lvclass">, "error out"=w1015:errorcluster)  [unwired: 14 in]
        n400 = call-dynamic "EnqueueMain.vi"("object in"=w1017, "Message"="CetoniReadCurrentSyringes", "error in (no error)"=w1015) -> ("object out"=w1016:refnum<class "Application.lvclass">, "error out"=w1014:errorcluster)  [unwired: 15 in]
      }
      event "Load and set latest": Value Change {
        n401 = event-data() -> ()  [unwired: 1 in, 2 out]
        n402 = call-dynamic "EnqueueMain.vi"("object in"=w1024, "Message"="CetoniConfigurationLoad") -> ("object out"=w1023:refnum<class "Application.lvclass">)  [unwired: 16 in, 1 out]
      }
      event "Save Current Configuration": Value Change {
        n403 = event-data() -> ()  [unwired: 1 in, 2 out]
        n404 = call-dynamic "EnqueueMain.vi"("object in"=w1027, "Message"="CetoniConfigurationWrite") -> ("object out"=w1026:refnum<class "Application.lvclass">)  [unwired: 16 in, 1 out]
      }
      event "Stop ALL Pumps": Value Change {
        n405 = event-data() -> ()  [unwired: 1 in, 1 out]
        n406 = call-dynamic "EnqueueMain.vi"("object in"=w1032, "Message"="CetoniStopAllSyringes", "error in (no error)"=w1028) -> ("object out"=w1031:refnum<class "Application.lvclass">, "error out"=w1029:errorcluster)  [unwired: 15 in]
      }
      event "Syringe (only for syringe helper)": Value Change {
        n407 = event-data() -> ()  [unwired: 1 in, 2 out]
        n408 = call-dynamic "BDSyringeHelper.vi"("object in"=refnum<class "CetoniPump.lvclass"> refnum, "Syringe"="Syringe (only for syringe helper)") -> ("output cluster"=→"Syringe Helper":T7)  [unwired: 15 in, 2 out]
      }
      event "Go to Level": Value Change {
        n409 = event-data() -> ()  [unwired: 1 in, 1 out]
        n410 = call-dynamic "EnqueueMain.vi"("object in"=w1042, "Message"="CetoniGoToLevel", "Message Data"="Go to Level", "error in (no error)"=w1038) -> ("object out"=w1041:refnum<class "Application.lvclass">, "error out"=w1039:errorcluster)  [unwired: 14 in]
      }
      event "Inject Error<Replace Me>": Value Change {
        # "#CodeNeeded - Send the appropriate message for this user interface event."
        n411 = event-data() -> ()  [unwired: 1 in, 1 out]
        n412 = call-dynamic "EnqueueMain.vi"("object in"=w1048, "Message"="InjectError", "Message Data"=errorcluster {"status"=TRUE, "code"=-8000, "source"="Injected Error"} ("error in (no error)"), "error in (no error)"=w1044) -> ("object out"=w1047:refnum<class "Application.lvclass">, "error out"=w1045:errorcluster)  [unwired: 14 in]
      }
      event Panel Close? {
        # "Send the 'Confirm Quit' message if the user closes the panel of the VI. Discard the event so the 'Confirm Quit' message has a chance to run."
        n413 = event-data() -> ()  [unwired: 1 in, 1 out]
        n414 = call-dynamic "EnqueueMain.vi"("object in"=w1050, "Message"="Confirm Quit", "error in (no error)"=w1052, "Priority Message? (F)"=TRUE) -> ("object out"=w1049:refnum<class "Application.lvclass">, "error out"=w1051:errorcluster)  [unwired: 14 in]
        n415 = event-data("Discard?"=TRUE) -> ()  [unwired: 1 in, 1 out]
      }
      event Application Instance Close {
        # "#CodeRecommended - When a project closes, all VIs within that project are aborted and leave memory. However, any code placed in this event frame is guaranteed to run to completion, so add any cleanup code that absolutely must happen here."
        n416 = event-data() -> ()  [unwired: 1 in, 1 out]
      }
      event "Exit": Value Change {
        n417 = event-data() -> ()  [unwired: 1 in, 1 out]
        n418 = call-dynamic "EnqueueMain.vi"("object in"=w1063, "Message"="Exit", "error in (no error)"=w1059, "Priority Message? (F)"=TRUE) -> ("object out"=w1062:refnum<class "Application.lvclass">, "error out"=w1058:errorcluster)  [unwired: 14 in]
      }
      event "ABORT": Value Change {
        w1065 = T16."Enabled" ("Disabled")
        n419 = event-data() -> ()  [unwired: 1 in, 1 out]
        n420 = call-dynamic "EnqueueMain.vi"("object in"=w1071, "Message"="Abort", "error in (no error)"=w1067, "Priority Message? (F)"=TRUE) -> ("object out"=w1070:refnum<class "Application.lvclass">, "error out"=w1066:errorcluster)  [unwired: 14 in]
        n421 = property on="Take HW Timed Image Pair" class="Bool"("DisabledEnum"=w1065) -> ()  [unwired: 2 in, 2 out]
        n422 = property on="Run Experiment" class="Bool"("DisabledEnum"=T16."Disabled" ("Disabled")) -> ()  [unwired: 2 in, 2 out]
        n423 = property on="Go Live" class="Bool (strict)"("DisabledEnum"=w1065) -> ()  [unwired: 2 in, 2 out]
      }
      event User Event {
        # "The Message Handling Loop processed an \"Exit\" message, which fired this event to stop the Event Handling Loop."
        n424 = event-data() -> ()  [unwired: 1 in, 1 out]
        n425 = call "IMAQ WindClose"("Close All Windows (False)"=TRUE, "error in (no error)"=w1073) -> ("error out"=w1072:errorcluster)  [unwired: 4 in]
      }
      event User Event {
        n426 = event-data() -> ("Message"=w1080:string, "Message Data"=w1077:variant)  [unwired: 1 in]
        n427 = case shown="\"UpdateHWTimed\"" w1080 {
          tunnel: w1079 -> [w1088 w1097 w1104 w1124 w1145 w1150]
          tunnel: [w1088 w1097 w1098 w1121 w1146 w1151] -> w1078
          tunnel: w1077 -> [w1087 _ w1106 w1125 w1147 w1152]
          frame "UpdateStatus" {
            n428 = Variant To Data(type="" ("Status"), Variant=w1087) -> (data=w1083:string)  [unwired: 1 in, 1 out]
            "Status" <- w1083
            n429 = feedback #1("" ("Status")) -> (w1084:string)
            n430 = Equal?(x=w1084, y=w1083) -> (x = y?=w1082:bool)
            n431 = feedback-in #1(w1083) -> ()
            n432 = case shown="False" w1082 {
              tunnel: w1083 -> [w1089 _]
              frame False {
                n433 = Get Date/Time In Seconds() -> (seconds since 1Jan1904=w1096:timestamp)
                n434 = Get Date/Time String(seconds (now)=w1096) -> (time string=w1093:string)  [unwired: 2 in, 1 out]
                n435 = feedback #2("" ("string")) -> (w1090:string)
                n436 = Concatenate Strings("\r", w1093, "\t", w1089, w1090) -> (w1092:string)
                "LOG" <- w1092
                n437 = feedback-in #2(w1092) -> ()
              }
              frame True {
              }
            }
          }
          frame Default {
          }
          frame "UpdateLive" {
            w1100 = 0 ("Window Number (0...15)")
            n438 = Variant To Data(error in=w1104, type=T22 refnum ("FreeRunningImage"), Variant=w1106) -> (data=w1103:T22, error out=w1102:errorcluster)
            n439 = call "IMAQ WindShow"("error in (no error)"=w1102, "Get/Set Status? (Set)"=FALSE, "Window Number (0...15)"=w1100) -> ("error out"=w1101:errorcluster, "Visible?"=w1099:bool)  [unwired: 3 in, 1 out]
            n440 = case shown="True" w1099 {
              tunnel: w1103 -> [_ w1114]
              tunnel: w1101 -> [w1108 w1113]
              tunnel: w1100 -> [_ w1112]
              tunnel: [w1108 w1110] -> w1098
              frame False {
              }
              frame True {
                n441 = call "IMAQ WindDraw"("Resize to Image Size? (Y)"=FALSE, "Window Number (0...15)"=w1112, "error in (no error)"=w1113, "Title"="Live Image", "Image"=w1114) -> ("error out"=w1111:errorcluster)  [unwired: 5 in, 1 out]
                n442 = call "IMAQ WindZoom 2"("Window Number (0...15)"=w1112, "error in (no error)"=w1111, "Zoom to Fit? (False)"=TRUE) -> ("error out"=w1110:errorcluster)  [unwired: 5 in, 3 out]
              }
            }
          }
          frame "UpdateHWTimed" {
            n443 = Variant To Data(error in=w1124, type=T22[] [] ("HWSyncedImages"), Variant=w1125) -> (data=w1123:T22[], error out=w1122:errorcluster)
            n444 = Build Array("Frame1" ("Title"), "Frame2" ("Title")) -> (w1117:string[])
            n445 = for {
              tunnel: w1123 -> [w1133] mode=indexing
              shift-right: [w1126] -> w1121
              shift-left: w1122 -> [w1132]
              tunnel: w1117 -> [w1128] mode=indexing
              i -> [w1130]
              n446 = Increment(x=w1130) -> (x+1=w1129:i32)
              n447 = call "IMAQ WindShow"("error in (no error)"=w1132, "Get/Set Status? (Set)"=FALSE, "Window Number (0...15)"=w1129) -> ("error out"=w1131:errorcluster, "Visible?"=w1127:bool)  [unwired: 3 in, 1 out]
              n448 = case shown="True" w1127 {
                tunnel: w1133 -> [_ w1140]
                tunnel: w1131 -> [w1135 w1139]
                tunnel: w1129 -> [_ w1137]
                tunnel: w1128 -> [_ w1138]
                tunnel: [w1135 w1136] -> w1126
                frame False {
                }
                frame True {
                  n449 = call "IMAQ WindDraw"("Resize to Image Size? (Y)"=FALSE, "Window Number (0...15)"=w1137, "error in (no error)"=w1139, "Title"=w1138, "Image"=w1140) -> ("error out"=w1136:errorcluster)  [unwired: 5 in, 1 out]
                }
              }
            }
          }
          frame "UpdateCoriolis" {
            n450 = Variant To Data(error in=w1145, type=T14 {"Cluster"={"Density_g_L"=0.0, "FLow(ul/min)"=0.0, "Temperature(C)"=0.0}, "current time"=timestamp(0 s since 1904-01-01)} ("Latest Data 2"), Variant=w1147) -> (data=w1143:T14, error out=w1146:errorcluster)
            "Coriolis  Data" <- w1143
            n451 = Unbundle By Name(w1143) -> ("Cluster"=→"Waveform Chart":T12)
          }
          frame "UpdateCetoni" {
            n452 = Variant To Data(error in=w1150, type=T2 [] ("Pump Array 2"), Variant=w1152) -> (data=→"Connected Pumps":T2, error out=w1151:errorcluster)
          }
        }
      }
      event "Run Experiment": Value Change {
        n453 = event-data() -> ()  [unwired: 1 in, 6 out]
        n454 = call-dynamic "EnqueueMain.vi"("object in"=w1156, "Message"="CoriolisFlushBuffer") -> ("object out"=w1157:refnum<class "Application.lvclass">)  [unwired: 16 in, 1 out]
        n455 = property on="Run Experiment" class="Bool"("DisabledEnum"=T16."Disabled and Grayed Out" ("Disabled")) -> ()  [unwired: 2 in, 2 out]
        n456 = property on="Go Live" class="Bool (strict)"("DisabledEnum"=T16."Disabled and Grayed Out" ("Disabled")) -> ()  [unwired: 2 in, 2 out]
        n457 = call-dynamic "EnqueueMain.vi"("object in"=w1157, "Message"="ExperimentStart") -> ("object out"=w1158:refnum<class "Application.lvclass">)  [unwired: 16 in, 1 out]
      }
    }
    n458 = call-dynamic "ErrorHandlerEventLoop.vi"("object in"=w882, "error in (no error)"=w884) -> ("object out"=w881:refnum<class "Application.lvclass">, "error out"=w883:errorcluster)  [unwired: 16 in]
  }
  n459 = disable-structure shown="Disabled" {
    frame Disabled {
      n460 = call "VisualizeTriggerTiming.vi"() -> ()  [unwired: 19 in, 1 out]
    }
    frame Enabled {
    }
  }
  n461 = Merge Errors(w8, w9) -> (w7:errorcluster)
  n462 = call-dynamic "CleanUp.vi"("object in"=w10, "error in (no error)"=w7) -> ("error out"=→"error out":errorcluster)  [unwired: 16 in, 1 out]
